vi "TestHarnessDPL-Saturday.vi"() -> ()   [LabVIEW 2024]
uses:
  <vilib>/Analysis/1siggen.llb/Ramp Pattern by Samples.vi
  <vilib>/measure/mamon.llb/Trigger Detection for 1 Channel.vi
  <vilib>/measure/mascope.llb/Transition Measurements 1 chan.vi
  <vilib>/Utility/file.llb/Write Delimited Spreadsheet (DBL).vi
  <vilib>/Analysis/1siggen.llb/Ramp Pattern by Delta.vi
  <vilib>/measure/mascope.llb/Amplitude and Levels 1 chan.vi
  <vilib>/Analysis/NI_AALBase.lvlib
  <userlib>/_OpenG.lib/time/time.llb/openg_time.lvlib
  <instrlib>/Detector SCPI/Detector SCPI.lvlib
  <instrlib>/Keithley 24XX/Keithley 24XX.lvlib
  <instrlib>/Keithley 648X Series/Keithley 648X Series.lvlib
  <vilib>/measure/NI_MAPro.lvlib
  <instrlib>/TTi TG5011a/TTi TG5011a.lvlib
panel:
  out "measurement info":T1 {"ref levels"."ref units" items=["absolute", "relative"]; "ref levels"."high ref level" format="%.2p"; "ref levels"."low ref level" format="%.2p"; "ref levels"."mid ref level" format="%.2p"; "end time" format="%.2p"; "start time" format="%.2p"}
  out "Searching":dbl[][](array[numeric])
  out "error out":errorcluster
  in  "Exit":bool
  in  "Measurement Mode":T2(tab)=enum."SweepCurrent (B2901)"
  in  "Heater":bool
  in  "DetectorData":T3(array[cluster])=[{"Name"="SWIR", "DAC Offset"=1870, "DAC StepsPerHGCount"=0.0}, {"Name"="MWIR", "DAC Offset"=688, "DAC StepsPerHGCount"=0.0}] {"DAC Offset" min=1 max=4095 step=1}
  in  "SPI Clock":i64=1000000
  in  "Oversample":i32=256 min=1 max=4096
  in  "Power":bool
  in  "Detector VISA":refnum<visa-resource-name>="Detector_EGSE"
  out "Detector Resource":refnum<visa-resource-name>="Detector_EGSE"
  out "Voltage (V)":dbl[](array[numeric])=[3.264, 0.0, 11.856, 11.996]
  out "Current (mA)":dbl[](array[numeric])=[0.0, 0.0, 12.8, -6.439]
  in  "ThrowAway":i32=100 min=1 max=10000
  out "Detector EGSE ID String":string="Aberystwyth University,Enfys Detector EGSE,#02.2,v0.5.0\r\n"
  in  "Current source":refnum<visa-resource-name>
  in  "Channel":i32 min=0 max=7
  in  "Collection":enum16{"Science", "Debug"}(ring)=enum."Debug"
  in  "Tolerance":dbl
  in  "Target Counts":i32 min=0 max=4095
  in  "Find Offset":bool
  out "Searching...":bool
  out "BoardTemperature":dbl=29.25
  in  "Tab Control":enum32{"Counts", "All Counts", "Temperature"}(tab)
  out "Counts":dbl(graph)=10.96875
  out "All Counts":T4(graph)={"subarray[0]"=1165.0625, "subarray[1]"=0.0, "subarray[2]"=4.4375, "subarray[3]"=4012.25, "subarray[4]"=2457.1875, "subarray[5]"=108.625, "subarray[6]"=1984.4375, "subarray[7]"=0.4375, "subarray[8]"=0.0}
  out "Temperature":dbl(graph)=29.25
  in  "ResetVDACstats":bool
  in  "Gain":u16(ring) items=["High", "Med", "Low"]
  in  "DAC Value":i32=688 min=0 max=4095 step=1
  in  "Detector":u16(ring)=1 items=["SWIR", "MWIR"]
  out "Peak-to-Peak (counts)":dbl=737.46875 format="%^.4g"
  out "rms (counts) 2":dbl=233.70780098659813 format="%^.4g"
  out "Mean Value (counts)":dbl=149.05195579441914
  out "Elapsed(uS)":i32=7203
  out "size":i32=439
  in  "Avg":i32=1 min=1 max=100
  in  "Pause":bool
  out "Waveform Graph":waveform(dbl)(graph)
  in  "Detector 3":u16(ring) items=["SWIR", "MWIR"]
  in  "Gain 3":u16(ring) items=["High", "Med", "Low"]
  in  "trigger slope":u16(ring)=1 items=["Falling Edge", "Rising Edge"]
  in  "level":dbl=2000.0 format="%#_13g"
  in  "hysteresis":dbl format="%.2p"
  out "Edge Time (ms)":dbl
  in  "SWIR/MWIR":bool=TRUE
  in  "SweepDataSelector":enum32{"Raw data", "SWIR"}(tab)
  in  "Export Button":bool
  out "Counts vs Channels":dbl[][](array[numeric])=[[1e-10, 128.75, 13.9375, 7.9375, 15.8125, 6.0, 7.25, 2030.9375, 4089.9375], [1.1220184543019634e-10, 129.9375, 14.0, 7.8125, 35.625, 6.0625, 7.1875, 2030.9375, 4089.9375], [1.2589254117941675e-10, 129.5, 13.9375, 8.0, 44.0625, 6.1875, 7.1875, 2030.9375, 4090.0], [1.4125375446227545e-10, 129.875, 14.0625, 7.9375, 17.3125, 6.125, 7.25, 2030.9375, 4089.875], [1.5848931924611137e-10, 129.9375, 14.0, 7.9375, 47.125, 6.125, 7.25, 2030.9375, 4089.9375], [1.778279410038923e-10, 130.125, 14.0625, 7.875, 32.875, 5.875, 7.1875, 2030.9375, 4090.0], [1.9952623149688797e-10, 129.5, 13.875, 7.875, 19.5, 5.8125, 7.3125, 2030.9375, 4089.9375], [2.23872113856834e-10, 130.0625, 13.9375, 7.9375, 12.625, 5.5625, 7.25, 2030.9375, 4090.0], [2.5118864315095804e-10, 130.8125, 14.0625, 7.9375, 20.3125, 6.0, 7.1875, 2030.9375, 4089.9375], [2.8183829312644536e-10, 129.75, 13.9375, 7.9375, 62.625, 6.25, 7.25, 2030.9375, 4089.9375], [3.1622776601683795e-10, 130.4375, 14.125, 7.9375, 53.75, 6.125, 7.25, 2030.9375, 4090.0], [3.5481338923357554e-10, 130.3125, 13.9375, 7.9375, 38.75, 5.9375, 7.1875, 2030.9375, 4089.875], [3.9810717055349735e-10, 129.8125, 14.0, 7.875, 45.75, 6.1875, 7.25, 2030.9375, 4090.0], [4.466835921509632e-10, 130.0, 14.0, 7.875, 76.4375, 6.4375, 7.25, 2030.9375, 4090.0], [5.011872336272724e-10, 130.625, 14.0625, 7.9375, 206.875, 9.25, 7.3125, 2030.9375, 4090.0], [5.623413251903491e-10, 130.3125, 13.9375, 7.875, 198.5, 8.9375, 7.25, 2030.9375, 4090.0], [6.309573444801933e-10, 130.0, 14.0625, 7.9375, 198.5625, 8.25, 7.25, 2030.9375, 4090.0], [7.07945784384138e-10, 130.5625, 14.125, 7.9375, 208.125, 8.4375, 7.3125, 2030.9375, 4089.875], [7.943282347242817e-10, 130.125, 13.9375, 7.875, 217.4375, 8.6875, 7.3125, 2030.9375, 4090.0], [8.912509381337457e-10, 130.0625, 13.9375, 7.9375, 206.875, 8.5625, 7.3125, 2030.9375, 4090.0], [1e-09, 129.9375, 13.9375, 7.875, 207.0, 8.4375, 7.375, 2030.9375, 4089.875], [1.1220184543019634e-09, 129.5, 13.9375, 7.875, 175.625, 8.125, 7.3125, 2030.9375, 4089.9375], [1.2589254117941673e-09, 130.75, 14.0, 7.875, 161.0, 7.9375, 7.3125, 2030.9375, 4090.0], [1.4125375446227544e-09, 130.0625, 14.0, 7.9375, 154.125, 7.75, 7.25, 2030.9375, 4089.9375], [1.5848931924611136e-09, 130.1875, 14.0, 7.875, 301.75, 10.5625, 7.375, 2030.9375, 4089.9375], [1.7782794100389228e-09, 130.875, 14.0625, 7.9375, 313.75, 10.8125, 7.4375, 2030.9375, 4089.875], [1.99526231496888e-09, 129.9375, 14.0, 7.8125, 299.75, 10.6875, 7.3125, 2030.9375, 4089.9375], [2.2387211385683402e-09, 129.875, 13.9375, 7.875, 298.1875, 10.375, 7.4375, 2030.9375, 4089.9375], [2.5118864315095803e-09, 130.75, 14.0, 7.9375, 441.125, 12.625, 7.375, 2030.875, 4090.0], [2.818382931264454e-09, 130.625, 14.0, 7.875, 490.4375, 13.375, 7.5, 2030.9375, 4089.9375], [3.1622776601683795e-09, 131.4375, 14.0625, 7.9375, 501.8125, 13.5625, 7.5, 2030.9375, 4090.0], [3.548133892335755e-09, 130.25, 14.0, 7.9375, 617.5, 15.3125, 7.625, 2030.9375, 4089.875], [3.981071705534974e-09, 129.6875, 13.9375, 7.875, 619.4375, 15.25, 7.5625, 2030.9375, 4090.0], [4.466835921509632e-09, 130.5, 14.0625, 7.875, 629.6875, 15.5, 7.5, 2030.9375, 4089.875], [5.011872336272724e-09, 130.875, 13.9375, 7.9375, 780.5625, 17.875, 7.5625, 2030.9375, 4090.0], [5.623413251903492e-09, 130.25, 14.125, 7.875, 917.1875, 20.125, 7.75, 2030.9375, 4090.0], [6.309573444801934e-09, 130.25, 14.0, 7.875, 931.5, 20.0625, 7.6875, 2030.9375, 4089.9375], [7.079457843841381e-09, 130.0, 14.0, 7.875, 1056.8125, 22.75, 7.8125, 2030.9375, 4090.0], [7.943282347242815e-09, 130.5625, 14.0625, 7.875, 1224.5, 24.8125, 7.8125, 2030.9375, 4090.0], [8.912509381337456e-09, 130.25, 14.0, 7.9375, 1380.75, 27.9375, 7.875, 2030.9375, 4089.9375], [1e-08, 130.125, 14.0, 7.9375, 1513.625, 29.9375, 8.0625, 2030.9375, 4089.875], [1.1220184543019634e-08, 130.625, 14.0, 7.9375, 1648.5, 34.5625, 8.125, 2030.9375, 4089.9375], [1.2589254117941673e-08, 131.0, 14.0625, 7.875, 1962.25, 41.625, 8.25, 2030.9375, 4090.0], [1.4125375446227542e-08, 130.875, 14.0625, 7.875, 2069.75, 44.625, 8.3125, 2030.9375, 4089.875], [1.5848931924611136e-08, 130.8125, 14.0625, 7.9375, 2404.875, 49.0, 8.4375, 2030.9375, 4089.9375], [1.7782794100389228e-08, 130.75, 14.125, 8.0, 2633.3125, 53.625, 8.6875, 2030.9375, 4090.125], [1.99526231496888e-08, 130.25, 14.0, 7.9375, 2979.375, 58.5, 8.8125, 2030.9375, 4090.0625], [2.2387211385683398e-08, 131.125, 14.0625, 7.9375, 3271.5, 64.5625, 8.9375, 2030.9375, 4089.9375], [2.51188643150958e-08, 131.4375, 14.125, 7.9375, 3737.375, 71.875, 9.25, 2030.9375, 4090.0], [2.8183829312644537e-08, 130.625, 14.0625, 7.875, 3908.375, 79.4375, 9.375, 2030.9375, 4089.9375], [3.16227766016838e-08, 130.875, 14.125, 7.8125, 3950.875, 88.5, 9.8125, 2030.9375, 4090.0625], [3.548133892335755e-08, 130.125, 14.0, 7.9375, 3963.5, 96.9375, 10.0, 2030.9375, 4090.0], [3.9810717055349736e-08, 130.375, 14.0, 7.875, 3980.25, 112.625, 10.25, 2030.9375, 4090.0625], [4.466835921509632e-08, 129.875, 14.0, 7.9375, 3991.125, 124.875, 10.6875, 2030.9375, 4090.0625], [5.0118723362727236e-08, 130.875, 14.0, 7.875, 3999.1875, 133.75, 11.1875, 2030.9375, 4090.0625], [5.623413251903492e-08, 130.25, 14.0, 8.0, 4007.9375, 147.125, 11.625, 2030.9375, 4090.0625], [6.309573444801934e-08, 130.75, 14.0625, 7.875, 4009.875, 168.1875, 12.1875, 2030.9375, 4090.0], [7.079457843841381e-08, 130.125, 13.9375, 7.875, 4010.0625, 187.6875, 12.875, 2030.9375, 4090.0], [7.943282347242817e-08, 130.1875, 14.0625, 7.9375, 4009.9375, 208.0625, 13.5625, 2030.9375, 4090.0], [8.912509381337456e-08, 130.75, 14.0625, 7.9375, 4010.0, 236.8125, 14.3125, 2030.9375, 4090.0], [1.0000000000000001e-07, 130.0, 14.0, 7.9375, 4010.0, 259.6875, 15.125, 2030.9375, 4089.9375], [1.1220184543019634e-07, 130.625, 14.125, 7.875, 4010.0, 288.4375, 16.125, 2030.9375, 4090.0625], [1.2589254117941672e-07, 130.6875, 14.0625, 8.0, 4009.9375, 326.375, 17.125, 2030.9375, 4090.0], [1.4125375446227544e-07, 130.5625, 14.0, 7.9375, 4010.0, 367.5625, 18.25, 2030.9375, 4090.0625], [1.5848931924611136e-07, 131.5, 14.0625, 7.875, 4010.0, 403.6875, 19.5, 2030.9375, 4090.0], [1.778279410038923e-07, 130.375, 14.0625, 7.9375, 4010.0, 457.875, 21.1875, 2030.9375, 4090.0], [1.9952623149688798e-07, 130.5625, 14.0, 8.0, 4010.0625, 512.6875, 22.875, 2030.9375, 4089.9375], [2.23872113856834e-07, 130.8125, 14.125, 7.9375, 4009.875, 571.875, 24.8125, 2030.9375, 4090.0], [2.51188643150958e-07, 130.125, 14.0, 7.9375, 4010.0625, 640.375, 26.9375, 2030.9375, 4090.125], [2.818382931264454e-07, 130.375, 14.0, 7.9375, 4010.0, 718.0625, 29.8125, 2030.9375, 4090.0], [3.1622776601683797e-07, 130.1875, 14.0625, 8.0, 4009.9375, 802.625, 34.125, 2030.9375, 4090.0625], [3.548133892335755e-07, 130.75, 14.0625, 7.9375, 4009.9375, 901.25, 39.375, 2030.9375, 4090.0625], [3.9810717055349735e-07, 130.4375, 14.0625, 7.9375, 4009.9375, 1014.0625, 43.8125, 2030.9375, 4089.9375], [4.4668359215096317e-07, 130.75, 14.125, 7.9375, 4009.8125, 1135.1875, 47.6875, 2030.9375, 4090.125], [5.011872336272724e-07, 130.5, 14.0625, 8.0, 4009.8125, 1270.3125, 52.0, 2030.9375, 4090.0625], [5.623413251903491e-07, 131.1875, 14.125, 7.9375, 4009.9375, 1418.75, 56.8125, 2030.9375, 4090.0], [6.309573444801933e-07, 130.625, 14.0, 7.9375, 4009.9375, 1591.875, 62.625, 2030.9375, 4090.0625], [7.07945784384138e-07, 130.25, 14.125, 7.9375, 4010.0, 1787.8125, 69.3125, 2031.0, 4090.0], [7.943282347242816e-07, 130.0625, 13.9375, 7.875, 4009.9375, 2000.625, 76.375, 2030.9375, 4090.0], [8.912509381337455e-07, 130.3125, 14.0625, 8.0625, 4009.8125, 2242.3125, 83.8125, 2030.9375, 4090.0625], [1e-06, 130.875, 14.0625, 7.9375, 4010.0, 2513.625, 92.6875, 2030.9375, 4090.0625], [1.1220184543019635e-06, 129.5625, 14.0, 8.0, 4009.8125, 2816.8125, 107.0, 2030.9375, 4090.0625], [1.2589254117941674e-06, 129.75, 14.0625, 7.9375, 4009.8125, 3157.6875, 118.25, 2030.9375, 4090.125], [1.4125375446227546e-06, 130.875, 14.0625, 7.875, 4009.9375, 3544.25, 128.75, 2030.9375, 4090.0625], [1.5848931924611137e-06, 130.125, 14.0625, 7.9375, 4009.9375, 3876.875, 140.5, 2030.9375, 4090.125], [1.7782794100389227e-06, 130.3125, 14.0625, 7.9375, 4009.75, 3932.25, 155.6875, 2030.9375, 4090.0], [1.9952623149688796e-06, 130.8125, 14.0625, 7.9375, 4009.75, 3955.5625, 177.8125, 2030.9375, 4090.1875], [2.23872113856834e-06, 129.9375, 14.0625, 8.0, 4009.875, 3970.6875, 198.0, 2030.9375, 4090.1875], [2.51188643150958e-06, 131.25, 14.1875, 8.0, 4009.875, 3982.125, 219.625, 2030.9375, 4090.125], [2.818382931264454e-06, 131.0, 14.125, 8.0, 4009.8125, 3992.0, 248.8125, 2030.9375, 4090.125], [3.1622776601683796e-06, 131.125, 14.0625, 8.0, 4009.9375, 4000.375, 272.8125, 2030.9375, 4090.0625], [3.548133892335755e-06, 131.3125, 14.125, 7.875, 4009.9375, 4006.3125, 308.25, 2030.9375, 4090.125], [3.981071705534973e-06, 130.875, 14.125, 7.9375, 4009.8125, 4006.3125, 343.3125, 2030.9375, 4090.1875], [4.466835921509632e-06, 130.5625, 14.125, 8.0, 4009.75, 4006.375, 385.0, 2030.9375, 4090.1875], [5.011872336272724e-06, 130.4375, 14.125, 8.0, 4009.875, 4006.3125, 431.1875, 2030.9375, 4090.1875], [5.623413251903491e-06, 130.25, 14.0625, 7.9375, 4010.0, 4006.3125, 481.875, 2030.9375, 4090.1875], [6.309573444801934e-06, 130.4375, 14.0625, 7.9375, 4009.9375, 4006.3125, 534.375, 2030.9375, 4090.125], [7.079457843841381e-06, 130.6875, 14.0625, 7.9375, 4009.875, 4006.3125, 601.1875, 2030.9375, 4090.125], [7.943282347242817e-06, 130.8125, 14.25, 8.0, 4009.875, 4006.3125, 671.5625, 2030.9375, 4090.1875], [8.912509381337456e-06, 130.6875, 14.0625, 8.0625, 4009.875, 4006.3125, 758.5, 2030.9375, 4090.125], [1e-05, 130.8125, 14.125, 8.0, 4009.75, 4006.3125, 847.125, 2030.9375, 4090.1875], [1.1220184543019633e-05, 131.25, 14.125, 8.0, 4009.8125, 4006.3125, 949.8125, 2030.9375, 4090.1875], [1.2589254117941673e-05, 130.625, 14.1875, 8.0, 4009.8125, 4006.3125, 1062.1875, 2030.9375, 4090.125], [1.4125375446227545e-05, 130.1875, 14.0625, 8.0, 4009.75, 4006.25, 1190.75, 2030.9375, 4090.1875], [1.5848931924611134e-05, 130.3125, 14.0625, 8.0, 4009.8125, 4006.3125, 1334.4375, 2030.9375, 4090.125], [1.778279410038923e-05, 130.625, 14.0625, 8.0, 4009.75, 4006.375, 1494.75, 2030.9375, 4090.1875], [1.99526231496888e-05, 130.75, 14.125, 8.0, 4009.8125, 4006.3125, 1672.4375, 2030.9375, 4090.25], [2.23872113856834e-05, 130.6875, 14.125, 8.0625, 4009.6875, 4006.375, 1877.3125, 2030.9375, 4090.25], [2.51188643150958e-05, 131.625, 14.1875, 8.0625, 4009.6875, 4006.3125, 2102.375, 2030.9375, 4090.1875], [2.818382931264454e-05, 129.875, 14.0625, 7.9375, 4009.75, 4006.25, 2358.0, 2030.9375, 4090.1875], [3.1622776601683795e-05, 130.1875, 14.125, 8.0, 4009.8125, 4006.3125, 2641.8125, 2030.9375, 4090.125], [3.5481338923357554e-05, 130.4375, 14.125, 8.0, 4009.75, 4006.375, 2960.6875, 2030.9375, 4090.1875], [3.9810717055349735e-05, 130.6875, 14.1875, 8.0, 4009.75, 4006.375, 3322.5, 2030.9375, 4090.125], [4.466835921509632e-05, 131.0, 14.125, 8.0, 4009.6875, 4006.375, 3719.875, 2031.0, 4090.1875], [5.011872336272724e-05, 130.75, 14.125, 8.0625, 4009.6875, 4006.375, 3911.125, 2030.9375, 4090.3125], [5.6234132519034914e-05, 130.875, 14.1875, 8.0625, 4009.625, 4006.375, 3946.3125, 2030.9375, 4090.25], [6.309573444801933e-05, 132.375, 14.1875, 8.0, 4009.625, 4006.3125, 3965.4375, 2031.0, 4090.3125], [7.079457843841381e-05, 131.1875, 14.25, 8.0, 4009.6875, 4006.375, 3979.0, 2030.9375, 4090.1875], [7.943282347242817e-05, 130.9375, 14.25, 8.0, 4009.625, 4006.375, 3990.25, 2031.0, 4090.1875], [8.912509381337456e-05, 130.9375, 14.25, 8.0625, 4009.5625, 4006.4375, 3999.8125, 2031.0, 4090.3125]]
  out "All Channel Data":cluster{dbl[], "output array":dbl[]}[](graph)=[{[1e-10, 1.1220184543019634e-10, 1.2589254117941675e-10, 1.4125375446227545e-10, 1.5848931924611137e-10, 1.778279410038923e-10, 1.9952623149688797e-10, 2.23872113856834e-10, 2.5118864315095804e-10, 2.8183829312644536e-10, 3.1622776601683795e-10, 3.5481338923357554e-10, 3.9810717055349735e-10, 4.466835921509632e-10, 5.011872336272724e-10, 5.623413251903491e-10, 6.309573444801933e-10, 7.07945784384138e-10, 7.943282347242817e-10, 8.912509381337457e-10, 1e-09, 1.1220184543019634e-09, 1.2589254117941673e-09, 1.4125375446227544e-09, 1.5848931924611136e-09, 1.7782794100389228e-09, 1.99526231496888e-09, 2.2387211385683402e-09, 2.5118864315095803e-09, 2.818382931264454e-09, 3.1622776601683795e-09, 3.548133892335755e-09, 3.981071705534974e-09, 4.466835921509632e-09, 5.011872336272724e-09, 5.623413251903492e-09, 6.309573444801934e-09, 7.079457843841381e-09, 7.943282347242815e-09, 8.912509381337456e-09, 1e-08, 1.1220184543019634e-08, 1.2589254117941673e-08, 1.4125375446227542e-08, 1.5848931924611136e-08, 1.7782794100389228e-08, 1.99526231496888e-08, 2.2387211385683398e-08, 2.51188643150958e-08, 2.8183829312644537e-08, 3.16227766016838e-08, 3.548133892335755e-08, 3.9810717055349736e-08, 4.466835921509632e-08, 5.0118723362727236e-08, 5.623413251903492e-08, 6.309573444801934e-08, 7.079457843841381e-08, 7.943282347242817e-08, 8.912509381337456e-08, 1.0000000000000001e-07, 1.1220184543019634e-07, 1.2589254117941672e-07, 1.4125375446227544e-07, 1.5848931924611136e-07, 1.778279410038923e-07, 1.9952623149688798e-07, 2.23872113856834e-07, 2.51188643150958e-07, 2.818382931264454e-07, 3.1622776601683797e-07, 3.548133892335755e-07, 3.9810717055349735e-07, 4.4668359215096317e-07, 5.011872336272724e-07, 5.623413251903491e-07, 6.309573444801933e-07, 7.07945784384138e-07, 7.943282347242816e-07, 8.912509381337455e-07, 1e-06, 1.1220184543019635e-06, 1.2589254117941674e-06, 1.4125375446227546e-06, 1.5848931924611137e-06, 1.7782794100389227e-06, 1.9952623149688796e-06, 2.23872113856834e-06, 2.51188643150958e-06, 2.818382931264454e-06, 3.1622776601683796e-06, 3.548133892335755e-06, 3.981071705534973e-06, 4.466835921509632e-06, 5.011872336272724e-06, 5.623413251903491e-06, 6.309573444801934e-06, 7.079457843841381e-06, 7.943282347242817e-06, 8.912509381337456e-06, 1e-05, 1.1220184543019633e-05, 1.2589254117941673e-05, 1.4125375446227545e-05, 1.5848931924611134e-05, 1.778279410038923e-05, 1.99526231496888e-05, 2.23872113856834e-05, 2.51188643150958e-05, 2.818382931264454e-05, 3.1622776601683795e-05, 3.5481338923357554e-05, 3.9810717055349735e-05, 4.466835921509632e-05, 5.011872336272724e-05, 5.6234132519034914e-05, 6.309573444801933e-05, 7.079457843841381e-05, 7.943282347242817e-05, 8.912509381337456e-05], "output array"=[15.8125, 35.625, 44.0625, 17.3125, 47.125, 32.875, 19.5, 12.625, 20.3125, 62.625, 53.75, 38.75, 45.75, 76.4375, 206.875, 198.5, 198.5625, 208.125, 217.4375, 206.875, 207.0, 175.625, 161.0, 154.125, 301.75, 313.75, 299.75, 298.1875, 441.125, 490.4375, 501.8125, 617.5, 619.4375, 629.6875, 780.5625, 917.1875, 931.5, 1056.8125, 1224.5, 1380.75, 1513.625, 1648.5, 1962.25, 2069.75, 2404.875, 2633.3125, 2979.375, 3271.5, 3737.375, 3908.375, 3950.875, 3963.5, 3980.25, 3991.125, 3999.1875, 4007.9375, 4009.875, 4010.0625, 4009.9375, 4010.0, 4010.0, 4010.0, 4009.9375, 4010.0, 4010.0, 4010.0, 4010.0625, 4009.875, 4010.0625, 4010.0, 4009.9375, 4009.9375, 4009.9375, 4009.8125, 4009.8125, 4009.9375, 4009.9375, 4010.0, 4009.9375, 4009.8125, 4010.0, 4009.8125, 4009.8125, 4009.9375, 4009.9375, 4009.75, 4009.75, 4009.875, 4009.875, 4009.8125, 4009.9375, 4009.9375, 4009.8125, 4009.75, 4009.875, 4010.0, 4009.9375, 4009.875, 4009.875, 4009.875, 4009.75, 4009.8125, 4009.8125, 4009.75, 4009.8125, 4009.75, 4009.8125, 4009.6875, 4009.6875, 4009.75, 4009.8125, 4009.75, 4009.75, 4009.6875, 4009.6875, 4009.625, 4009.625, 4009.6875, 4009.625, 4009.5625]}, {[1e-10, 1.1220184543019634e-10, 1.2589254117941675e-10, 1.4125375446227545e-10, 1.5848931924611137e-10, 1.778279410038923e-10, 1.9952623149688797e-10, 2.23872113856834e-10, 2.5118864315095804e-10, 2.8183829312644536e-10, 3.1622776601683795e-10, 3.5481338923357554e-10, 3.9810717055349735e-10, 4.466835921509632e-10, 5.011872336272724e-10, 5.623413251903491e-10, 6.309573444801933e-10, 7.07945784384138e-10, 7.943282347242817e-10, 8.912509381337457e-10, 1e-09, 1.1220184543019634e-09, 1.2589254117941673e-09, 1.4125375446227544e-09, 1.5848931924611136e-09, 1.7782794100389228e-09, 1.99526231496888e-09, 2.2387211385683402e-09, 2.5118864315095803e-09, 2.818382931264454e-09, 3.1622776601683795e-09, 3.548133892335755e-09, 3.981071705534974e-09, 4.466835921509632e-09, 5.011872336272724e-09, 5.623413251903492e-09, 6.309573444801934e-09, 7.079457843841381e-09, 7.943282347242815e-09, 8.912509381337456e-09, 1e-08, 1.1220184543019634e-08, 1.2589254117941673e-08, 1.4125375446227542e-08, 1.5848931924611136e-08, 1.7782794100389228e-08, 1.99526231496888e-08, 2.2387211385683398e-08, 2.51188643150958e-08, 2.8183829312644537e-08, 3.16227766016838e-08, 3.548133892335755e-08, 3.9810717055349736e-08, 4.466835921509632e-08, 5.0118723362727236e-08, 5.623413251903492e-08, 6.309573444801934e-08, 7.079457843841381e-08, 7.943282347242817e-08, 8.912509381337456e-08, 1.0000000000000001e-07, 1.1220184543019634e-07, 1.2589254117941672e-07, 1.4125375446227544e-07, 1.5848931924611136e-07, 1.778279410038923e-07, 1.9952623149688798e-07, 2.23872113856834e-07, 2.51188643150958e-07, 2.818382931264454e-07, 3.1622776601683797e-07, 3.548133892335755e-07, 3.9810717055349735e-07, 4.4668359215096317e-07, 5.011872336272724e-07, 5.623413251903491e-07, 6.309573444801933e-07, 7.07945784384138e-07, 7.943282347242816e-07, 8.912509381337455e-07, 1e-06, 1.1220184543019635e-06, 1.2589254117941674e-06, 1.4125375446227546e-06, 1.5848931924611137e-06, 1.7782794100389227e-06, 1.9952623149688796e-06, 2.23872113856834e-06, 2.51188643150958e-06, 2.818382931264454e-06, 3.1622776601683796e-06, 3.548133892335755e-06, 3.981071705534973e-06, 4.466835921509632e-06, 5.011872336272724e-06, 5.623413251903491e-06, 6.309573444801934e-06, 7.079457843841381e-06, 7.943282347242817e-06, 8.912509381337456e-06, 1e-05, 1.1220184543019633e-05, 1.2589254117941673e-05, 1.4125375446227545e-05, 1.5848931924611134e-05, 1.778279410038923e-05, 1.99526231496888e-05, 2.23872113856834e-05, 2.51188643150958e-05, 2.818382931264454e-05, 3.1622776601683795e-05, 3.5481338923357554e-05, 3.9810717055349735e-05, 4.466835921509632e-05, 5.011872336272724e-05, 5.6234132519034914e-05, 6.309573444801933e-05, 7.079457843841381e-05, 7.943282347242817e-05, 8.912509381337456e-05], "output array"=[6.0, 6.0625, 6.1875, 6.125, 6.125, 5.875, 5.8125, 5.5625, 6.0, 6.25, 6.125, 5.9375, 6.1875, 6.4375, 9.25, 8.9375, 8.25, 8.4375, 8.6875, 8.5625, 8.4375, 8.125, 7.9375, 7.75, 10.5625, 10.8125, 10.6875, 10.375, 12.625, 13.375, 13.5625, 15.3125, 15.25, 15.5, 17.875, 20.125, 20.0625, 22.75, 24.8125, 27.9375, 29.9375, 34.5625, 41.625, 44.625, 49.0, 53.625, 58.5, 64.5625, 71.875, 79.4375, 88.5, 96.9375, 112.625, 124.875, 133.75, 147.125, 168.1875, 187.6875, 208.0625, 236.8125, 259.6875, 288.4375, 326.375, 367.5625, 403.6875, 457.875, 512.6875, 571.875, 640.375, 718.0625, 802.625, 901.25, 1014.0625, 1135.1875, 1270.3125, 1418.75, 1591.875, 1787.8125, 2000.625, 2242.3125, 2513.625, 2816.8125, 3157.6875, 3544.25, 3876.875, 3932.25, 3955.5625, 3970.6875, 3982.125, 3992.0, 4000.375, 4006.3125, 4006.3125, 4006.375, 4006.3125, 4006.3125, 4006.3125, 4006.3125, 4006.3125, 4006.3125, 4006.3125, 4006.3125, 4006.3125, 4006.25, 4006.3125, 4006.375, 4006.3125, 4006.375, 4006.3125, 4006.25, 4006.3125, 4006.375, 4006.375, 4006.375, 4006.375, 4006.375, 4006.3125, 4006.375, 4006.375, 4006.4375]}, {[1e-10, 1.1220184543019634e-10, 1.2589254117941675e-10, 1.4125375446227545e-10, 1.5848931924611137e-10, 1.778279410038923e-10, 1.9952623149688797e-10, 2.23872113856834e-10, 2.5118864315095804e-10, 2.8183829312644536e-10, 3.1622776601683795e-10, 3.5481338923357554e-10, 3.9810717055349735e-10, 4.466835921509632e-10, 5.011872336272724e-10, 5.623413251903491e-10, 6.309573444801933e-10, 7.07945784384138e-10, 7.943282347242817e-10, 8.912509381337457e-10, 1e-09, 1.1220184543019634e-09, 1.2589254117941673e-09, 1.4125375446227544e-09, 1.5848931924611136e-09, 1.7782794100389228e-09, 1.99526231496888e-09, 2.2387211385683402e-09, 2.5118864315095803e-09, 2.818382931264454e-09, 3.1622776601683795e-09, 3.548133892335755e-09, 3.981071705534974e-09, 4.466835921509632e-09, 5.011872336272724e-09, 5.623413251903492e-09, 6.309573444801934e-09, 7.079457843841381e-09, 7.943282347242815e-09, 8.912509381337456e-09, 1e-08, 1.1220184543019634e-08, 1.2589254117941673e-08, 1.4125375446227542e-08, 1.5848931924611136e-08, 1.7782794100389228e-08, 1.99526231496888e-08, 2.2387211385683398e-08, 2.51188643150958e-08, 2.8183829312644537e-08, 3.16227766016838e-08, 3.548133892335755e-08, 3.9810717055349736e-08, 4.466835921509632e-08, 5.0118723362727236e-08, 5.623413251903492e-08, 6.309573444801934e-08, 7.079457843841381e-08, 7.943282347242817e-08, 8.912509381337456e-08, 1.0000000000000001e-07, 1.1220184543019634e-07, 1.2589254117941672e-07, 1.4125375446227544e-07, 1.5848931924611136e-07, 1.778279410038923e-07, 1.9952623149688798e-07, 2.23872113856834e-07, 2.51188643150958e-07, 2.818382931264454e-07, 3.1622776601683797e-07, 3.548133892335755e-07, 3.9810717055349735e-07, 4.4668359215096317e-07, 5.011872336272724e-07, 5.623413251903491e-07, 6.309573444801933e-07, 7.07945784384138e-07, 7.943282347242816e-07, 8.912509381337455e-07, 1e-06, 1.1220184543019635e-06, 1.2589254117941674e-06, 1.4125375446227546e-06, 1.5848931924611137e-06, 1.7782794100389227e-06, 1.9952623149688796e-06, 2.23872113856834e-06, 2.51188643150958e-06, 2.818382931264454e-06, 3.1622776601683796e-06, 3.548133892335755e-06, 3.981071705534973e-06, 4.466835921509632e-06, 5.011872336272724e-06, 5.623413251903491e-06, 6.309573444801934e-06, 7.079457843841381e-06, 7.943282347242817e-06, 8.912509381337456e-06, 1e-05, 1.1220184543019633e-05, 1.2589254117941673e-05, 1.4125375446227545e-05, 1.5848931924611134e-05, 1.778279410038923e-05, 1.99526231496888e-05, 2.23872113856834e-05, 2.51188643150958e-05, 2.818382931264454e-05, 3.1622776601683795e-05, 3.5481338923357554e-05, 3.9810717055349735e-05, 4.466835921509632e-05, 5.011872336272724e-05, 5.6234132519034914e-05, 6.309573444801933e-05, 7.079457843841381e-05, 7.943282347242817e-05, 8.912509381337456e-05], "output array"=[7.25, 7.1875, 7.1875, 7.25, 7.25, 7.1875, 7.3125, 7.25, 7.1875, 7.25, 7.25, 7.1875, 7.25, 7.25, 7.3125, 7.25, 7.25, 7.3125, 7.3125, 7.3125, 7.375, 7.3125, 7.3125, 7.25, 7.375, 7.4375, 7.3125, 7.4375, 7.375, 7.5, 7.5, 7.625, 7.5625, 7.5, 7.5625, 7.75, 7.6875, 7.8125, 7.8125, 7.875, 8.0625, 8.125, 8.25, 8.3125, 8.4375, 8.6875, 8.8125, 8.9375, 9.25, 9.375, 9.8125, 10.0, 10.25, 10.6875, 11.1875, 11.625, 12.1875, 12.875, 13.5625, 14.3125, 15.125, 16.125, 17.125, 18.25, 19.5, 21.1875, 22.875, 24.8125, 26.9375, 29.8125, 34.125, 39.375, 43.8125, 47.6875, 52.0, 56.8125, 62.625, 69.3125, 76.375, 83.8125, 92.6875, 107.0, 118.25, 128.75, 140.5, 155.6875, 177.8125, 198.0, 219.625, 248.8125, 272.8125, 308.25, 343.3125, 385.0, 431.1875, 481.875, 534.375, 601.1875, 671.5625, 758.5, 847.125, 949.8125, 1062.1875, 1190.75, 1334.4375, 1494.75, 1672.4375, 1877.3125, 2102.375, 2358.0, 2641.8125, 2960.6875, 3322.5, 3719.875, 3911.125, 3946.3125, 3965.4375, 3979.0, 3990.25, 3999.8125]}]
  in  "ISweep":bool
  in  "NPoints":i32=10 min=10 max=10000 step=1
  in  "MaxCurrent":dbl=1e-11 min=1e-11 max=1e-06
  in  "MinCurrent":dbl=1e-10 min=-10.0 max=10.0
  in  "DecadeSweep":bool=TRUE
  in  "milliseconds stabilisation":u32=10
  in  "SuperAverage":i32=1 min=1 max=100
  in  "NPointsPerDecade":u16(ring)=3 items=["1", "3", "9", "20"]
  in  "Tab Control 2":enum32{"Raw Data", "Plot"}(tab)
  in  "ExportData":bool
  out "Counts vs Channels 2":dbl[][](array[numeric])=[[1e-10, 128.75, 13.9375, 7.9375, 15.8125, 6.0, 7.25, 2030.9375, 4089.9375], [1.1220184543019634e-10, 129.9375, 14.0, 7.8125, 35.625, 6.0625, 7.1875, 2030.9375, 4089.9375], [1.2589254117941675e-10, 129.5, 13.9375, 8.0, 44.0625, 6.1875, 7.1875, 2030.9375, 4090.0], [1.4125375446227545e-10, 129.875, 14.0625, 7.9375, 17.3125, 6.125, 7.25, 2030.9375, 4089.875], [1.5848931924611137e-10, 129.9375, 14.0, 7.9375, 47.125, 6.125, 7.25, 2030.9375, 4089.9375], [1.778279410038923e-10, 130.125, 14.0625, 7.875, 32.875, 5.875, 7.1875, 2030.9375, 4090.0], [1.9952623149688797e-10, 129.5, 13.875, 7.875, 19.5, 5.8125, 7.3125, 2030.9375, 4089.9375], [2.23872113856834e-10, 130.0625, 13.9375, 7.9375, 12.625, 5.5625, 7.25, 2030.9375, 4090.0], [2.5118864315095804e-10, 130.8125, 14.0625, 7.9375, 20.3125, 6.0, 7.1875, 2030.9375, 4089.9375], [2.8183829312644536e-10, 129.75, 13.9375, 7.9375, 62.625, 6.25, 7.25, 2030.9375, 4089.9375], [3.1622776601683795e-10, 130.4375, 14.125, 7.9375, 53.75, 6.125, 7.25, 2030.9375, 4090.0], [3.5481338923357554e-10, 130.3125, 13.9375, 7.9375, 38.75, 5.9375, 7.1875, 2030.9375, 4089.875], [3.9810717055349735e-10, 129.8125, 14.0, 7.875, 45.75, 6.1875, 7.25, 2030.9375, 4090.0], [4.466835921509632e-10, 130.0, 14.0, 7.875, 76.4375, 6.4375, 7.25, 2030.9375, 4090.0], [5.011872336272724e-10, 130.625, 14.0625, 7.9375, 206.875, 9.25, 7.3125, 2030.9375, 4090.0], [5.623413251903491e-10, 130.3125, 13.9375, 7.875, 198.5, 8.9375, 7.25, 2030.9375, 4090.0], [6.309573444801933e-10, 130.0, 14.0625, 7.9375, 198.5625, 8.25, 7.25, 2030.9375, 4090.0], [7.07945784384138e-10, 130.5625, 14.125, 7.9375, 208.125, 8.4375, 7.3125, 2030.9375, 4089.875], [7.943282347242817e-10, 130.125, 13.9375, 7.875, 217.4375, 8.6875, 7.3125, 2030.9375, 4090.0], [8.912509381337457e-10, 130.0625, 13.9375, 7.9375, 206.875, 8.5625, 7.3125, 2030.9375, 4090.0], [1e-09, 129.9375, 13.9375, 7.875, 207.0, 8.4375, 7.375, 2030.9375, 4089.875], [1.1220184543019634e-09, 129.5, 13.9375, 7.875, 175.625, 8.125, 7.3125, 2030.9375, 4089.9375], [1.2589254117941673e-09, 130.75, 14.0, 7.875, 161.0, 7.9375, 7.3125, 2030.9375, 4090.0], [1.4125375446227544e-09, 130.0625, 14.0, 7.9375, 154.125, 7.75, 7.25, 2030.9375, 4089.9375], [1.5848931924611136e-09, 130.1875, 14.0, 7.875, 301.75, 10.5625, 7.375, 2030.9375, 4089.9375], [1.7782794100389228e-09, 130.875, 14.0625, 7.9375, 313.75, 10.8125, 7.4375, 2030.9375, 4089.875], [1.99526231496888e-09, 129.9375, 14.0, 7.8125, 299.75, 10.6875, 7.3125, 2030.9375, 4089.9375], [2.2387211385683402e-09, 129.875, 13.9375, 7.875, 298.1875, 10.375, 7.4375, 2030.9375, 4089.9375], [2.5118864315095803e-09, 130.75, 14.0, 7.9375, 441.125, 12.625, 7.375, 2030.875, 4090.0], [2.818382931264454e-09, 130.625, 14.0, 7.875, 490.4375, 13.375, 7.5, 2030.9375, 4089.9375], [3.1622776601683795e-09, 131.4375, 14.0625, 7.9375, 501.8125, 13.5625, 7.5, 2030.9375, 4090.0], [3.548133892335755e-09, 130.25, 14.0, 7.9375, 617.5, 15.3125, 7.625, 2030.9375, 4089.875], [3.981071705534974e-09, 129.6875, 13.9375, 7.875, 619.4375, 15.25, 7.5625, 2030.9375, 4090.0], [4.466835921509632e-09, 130.5, 14.0625, 7.875, 629.6875, 15.5, 7.5, 2030.9375, 4089.875], [5.011872336272724e-09, 130.875, 13.9375, 7.9375, 780.5625, 17.875, 7.5625, 2030.9375, 4090.0], [5.623413251903492e-09, 130.25, 14.125, 7.875, 917.1875, 20.125, 7.75, 2030.9375, 4090.0], [6.309573444801934e-09, 130.25, 14.0, 7.875, 931.5, 20.0625, 7.6875, 2030.9375, 4089.9375], [7.079457843841381e-09, 130.0, 14.0, 7.875, 1056.8125, 22.75, 7.8125, 2030.9375, 4090.0], [7.943282347242815e-09, 130.5625, 14.0625, 7.875, 1224.5, 24.8125, 7.8125, 2030.9375, 4090.0], [8.912509381337456e-09, 130.25, 14.0, 7.9375, 1380.75, 27.9375, 7.875, 2030.9375, 4089.9375], [1e-08, 130.125, 14.0, 7.9375, 1513.625, 29.9375, 8.0625, 2030.9375, 4089.875], [1.1220184543019634e-08, 130.625, 14.0, 7.9375, 1648.5, 34.5625, 8.125, 2030.9375, 4089.9375], [1.2589254117941673e-08, 131.0, 14.0625, 7.875, 1962.25, 41.625, 8.25, 2030.9375, 4090.0], [1.4125375446227542e-08, 130.875, 14.0625, 7.875, 2069.75, 44.625, 8.3125, 2030.9375, 4089.875], [1.5848931924611136e-08, 130.8125, 14.0625, 7.9375, 2404.875, 49.0, 8.4375, 2030.9375, 4089.9375], [1.7782794100389228e-08, 130.75, 14.125, 8.0, 2633.3125, 53.625, 8.6875, 2030.9375, 4090.125], [1.99526231496888e-08, 130.25, 14.0, 7.9375, 2979.375, 58.5, 8.8125, 2030.9375, 4090.0625], [2.2387211385683398e-08, 131.125, 14.0625, 7.9375, 3271.5, 64.5625, 8.9375, 2030.9375, 4089.9375], [2.51188643150958e-08, 131.4375, 14.125, 7.9375, 3737.375, 71.875, 9.25, 2030.9375, 4090.0], [2.8183829312644537e-08, 130.625, 14.0625, 7.875, 3908.375, 79.4375, 9.375, 2030.9375, 4089.9375], [3.16227766016838e-08, 130.875, 14.125, 7.8125, 3950.875, 88.5, 9.8125, 2030.9375, 4090.0625], [3.548133892335755e-08, 130.125, 14.0, 7.9375, 3963.5, 96.9375, 10.0, 2030.9375, 4090.0], [3.9810717055349736e-08, 130.375, 14.0, 7.875, 3980.25, 112.625, 10.25, 2030.9375, 4090.0625], [4.466835921509632e-08, 129.875, 14.0, 7.9375, 3991.125, 124.875, 10.6875, 2030.9375, 4090.0625], [5.0118723362727236e-08, 130.875, 14.0, 7.875, 3999.1875, 133.75, 11.1875, 2030.9375, 4090.0625], [5.623413251903492e-08, 130.25, 14.0, 8.0, 4007.9375, 147.125, 11.625, 2030.9375, 4090.0625], [6.309573444801934e-08, 130.75, 14.0625, 7.875, 4009.875, 168.1875, 12.1875, 2030.9375, 4090.0], [7.079457843841381e-08, 130.125, 13.9375, 7.875, 4010.0625, 187.6875, 12.875, 2030.9375, 4090.0], [7.943282347242817e-08, 130.1875, 14.0625, 7.9375, 4009.9375, 208.0625, 13.5625, 2030.9375, 4090.0], [8.912509381337456e-08, 130.75, 14.0625, 7.9375, 4010.0, 236.8125, 14.3125, 2030.9375, 4090.0], [1.0000000000000001e-07, 130.0, 14.0, 7.9375, 4010.0, 259.6875, 15.125, 2030.9375, 4089.9375], [1.1220184543019634e-07, 130.625, 14.125, 7.875, 4010.0, 288.4375, 16.125, 2030.9375, 4090.0625], [1.2589254117941672e-07, 130.6875, 14.0625, 8.0, 4009.9375, 326.375, 17.125, 2030.9375, 4090.0], [1.4125375446227544e-07, 130.5625, 14.0, 7.9375, 4010.0, 367.5625, 18.25, 2030.9375, 4090.0625], [1.5848931924611136e-07, 131.5, 14.0625, 7.875, 4010.0, 403.6875, 19.5, 2030.9375, 4090.0], [1.778279410038923e-07, 130.375, 14.0625, 7.9375, 4010.0, 457.875, 21.1875, 2030.9375, 4090.0], [1.9952623149688798e-07, 130.5625, 14.0, 8.0, 4010.0625, 512.6875, 22.875, 2030.9375, 4089.9375], [2.23872113856834e-07, 130.8125, 14.125, 7.9375, 4009.875, 571.875, 24.8125, 2030.9375, 4090.0], [2.51188643150958e-07, 130.125, 14.0, 7.9375, 4010.0625, 640.375, 26.9375, 2030.9375, 4090.125], [2.818382931264454e-07, 130.375, 14.0, 7.9375, 4010.0, 718.0625, 29.8125, 2030.9375, 4090.0], [3.1622776601683797e-07, 130.1875, 14.0625, 8.0, 4009.9375, 802.625, 34.125, 2030.9375, 4090.0625], [3.548133892335755e-07, 130.75, 14.0625, 7.9375, 4009.9375, 901.25, 39.375, 2030.9375, 4090.0625], [3.9810717055349735e-07, 130.4375, 14.0625, 7.9375, 4009.9375, 1014.0625, 43.8125, 2030.9375, 4089.9375], [4.4668359215096317e-07, 130.75, 14.125, 7.9375, 4009.8125, 1135.1875, 47.6875, 2030.9375, 4090.125], [5.011872336272724e-07, 130.5, 14.0625, 8.0, 4009.8125, 1270.3125, 52.0, 2030.9375, 4090.0625], [5.623413251903491e-07, 131.1875, 14.125, 7.9375, 4009.9375, 1418.75, 56.8125, 2030.9375, 4090.0], [6.309573444801933e-07, 130.625, 14.0, 7.9375, 4009.9375, 1591.875, 62.625, 2030.9375, 4090.0625], [7.07945784384138e-07, 130.25, 14.125, 7.9375, 4010.0, 1787.8125, 69.3125, 2031.0, 4090.0], [7.943282347242816e-07, 130.0625, 13.9375, 7.875, 4009.9375, 2000.625, 76.375, 2030.9375, 4090.0], [8.912509381337455e-07, 130.3125, 14.0625, 8.0625, 4009.8125, 2242.3125, 83.8125, 2030.9375, 4090.0625], [1e-06, 130.875, 14.0625, 7.9375, 4010.0, 2513.625, 92.6875, 2030.9375, 4090.0625], [1.1220184543019635e-06, 129.5625, 14.0, 8.0, 4009.8125, 2816.8125, 107.0, 2030.9375, 4090.0625], [1.2589254117941674e-06, 129.75, 14.0625, 7.9375, 4009.8125, 3157.6875, 118.25, 2030.9375, 4090.125], [1.4125375446227546e-06, 130.875, 14.0625, 7.875, 4009.9375, 3544.25, 128.75, 2030.9375, 4090.0625], [1.5848931924611137e-06, 130.125, 14.0625, 7.9375, 4009.9375, 3876.875, 140.5, 2030.9375, 4090.125], [1.7782794100389227e-06, 130.3125, 14.0625, 7.9375, 4009.75, 3932.25, 155.6875, 2030.9375, 4090.0], [1.9952623149688796e-06, 130.8125, 14.0625, 7.9375, 4009.75, 3955.5625, 177.8125, 2030.9375, 4090.1875], [2.23872113856834e-06, 129.9375, 14.0625, 8.0, 4009.875, 3970.6875, 198.0, 2030.9375, 4090.1875], [2.51188643150958e-06, 131.25, 14.1875, 8.0, 4009.875, 3982.125, 219.625, 2030.9375, 4090.125], [2.818382931264454e-06, 131.0, 14.125, 8.0, 4009.8125, 3992.0, 248.8125, 2030.9375, 4090.125], [3.1622776601683796e-06, 131.125, 14.0625, 8.0, 4009.9375, 4000.375, 272.8125, 2030.9375, 4090.0625], [3.548133892335755e-06, 131.3125, 14.125, 7.875, 4009.9375, 4006.3125, 308.25, 2030.9375, 4090.125], [3.981071705534973e-06, 130.875, 14.125, 7.9375, 4009.8125, 4006.3125, 343.3125, 2030.9375, 4090.1875], [4.466835921509632e-06, 130.5625, 14.125, 8.0, 4009.75, 4006.375, 385.0, 2030.9375, 4090.1875], [5.011872336272724e-06, 130.4375, 14.125, 8.0, 4009.875, 4006.3125, 431.1875, 2030.9375, 4090.1875], [5.623413251903491e-06, 130.25, 14.0625, 7.9375, 4010.0, 4006.3125, 481.875, 2030.9375, 4090.1875], [6.309573444801934e-06, 130.4375, 14.0625, 7.9375, 4009.9375, 4006.3125, 534.375, 2030.9375, 4090.125], [7.079457843841381e-06, 130.6875, 14.0625, 7.9375, 4009.875, 4006.3125, 601.1875, 2030.9375, 4090.125], [7.943282347242817e-06, 130.8125, 14.25, 8.0, 4009.875, 4006.3125, 671.5625, 2030.9375, 4090.1875], [8.912509381337456e-06, 130.6875, 14.0625, 8.0625, 4009.875, 4006.3125, 758.5, 2030.9375, 4090.125], [1e-05, 130.8125, 14.125, 8.0, 4009.75, 4006.3125, 847.125, 2030.9375, 4090.1875], [1.1220184543019633e-05, 131.25, 14.125, 8.0, 4009.8125, 4006.3125, 949.8125, 2030.9375, 4090.1875], [1.2589254117941673e-05, 130.625, 14.1875, 8.0, 4009.8125, 4006.3125, 1062.1875, 2030.9375, 4090.125], [1.4125375446227545e-05, 130.1875, 14.0625, 8.0, 4009.75, 4006.25, 1190.75, 2030.9375, 4090.1875], [1.5848931924611134e-05, 130.3125, 14.0625, 8.0, 4009.8125, 4006.3125, 1334.4375, 2030.9375, 4090.125], [1.778279410038923e-05, 130.625, 14.0625, 8.0, 4009.75, 4006.375, 1494.75, 2030.9375, 4090.1875], [1.99526231496888e-05, 130.75, 14.125, 8.0, 4009.8125, 4006.3125, 1672.4375, 2030.9375, 4090.25], [2.23872113856834e-05, 130.6875, 14.125, 8.0625, 4009.6875, 4006.375, 1877.3125, 2030.9375, 4090.25], [2.51188643150958e-05, 131.625, 14.1875, 8.0625, 4009.6875, 4006.3125, 2102.375, 2030.9375, 4090.1875], [2.818382931264454e-05, 129.875, 14.0625, 7.9375, 4009.75, 4006.25, 2358.0, 2030.9375, 4090.1875], [3.1622776601683795e-05, 130.1875, 14.125, 8.0, 4009.8125, 4006.3125, 2641.8125, 2030.9375, 4090.125], [3.5481338923357554e-05, 130.4375, 14.125, 8.0, 4009.75, 4006.375, 2960.6875, 2030.9375, 4090.1875], [3.9810717055349735e-05, 130.6875, 14.1875, 8.0, 4009.75, 4006.375, 3322.5, 2030.9375, 4090.125], [4.466835921509632e-05, 131.0, 14.125, 8.0, 4009.6875, 4006.375, 3719.875, 2031.0, 4090.1875], [5.011872336272724e-05, 130.75, 14.125, 8.0625, 4009.6875, 4006.375, 3911.125, 2030.9375, 4090.3125], [5.6234132519034914e-05, 130.875, 14.1875, 8.0625, 4009.625, 4006.375, 3946.3125, 2030.9375, 4090.25], [6.309573444801933e-05, 132.375, 14.1875, 8.0, 4009.625, 4006.3125, 3965.4375, 2031.0, 4090.3125], [7.079457843841381e-05, 131.1875, 14.25, 8.0, 4009.6875, 4006.375, 3979.0, 2030.9375, 4090.1875], [7.943282347242817e-05, 130.9375, 14.25, 8.0, 4009.625, 4006.375, 3990.25, 2031.0, 4090.1875], [8.912509381337456e-05, 130.9375, 14.25, 8.0625, 4009.5625, 4006.4375, 3999.8125, 2031.0, 4090.3125]]
  out "All Channel Data 2":cluster{dbl[], "output array":dbl[]}[](graph)=[{[1e-10, 1.1220184543019634e-10, 1.2589254117941675e-10, 1.4125375446227545e-10, 1.5848931924611137e-10, 1.778279410038923e-10, 1.9952623149688797e-10, 2.23872113856834e-10, 2.5118864315095804e-10, 2.8183829312644536e-10, 3.1622776601683795e-10, 3.5481338923357554e-10, 3.9810717055349735e-10, 4.466835921509632e-10, 5.011872336272724e-10, 5.623413251903491e-10, 6.309573444801933e-10, 7.07945784384138e-10, 7.943282347242817e-10, 8.912509381337457e-10, 1e-09, 1.1220184543019634e-09, 1.2589254117941673e-09, 1.4125375446227544e-09, 1.5848931924611136e-09, 1.7782794100389228e-09, 1.99526231496888e-09, 2.2387211385683402e-09, 2.5118864315095803e-09, 2.818382931264454e-09, 3.1622776601683795e-09, 3.548133892335755e-09, 3.981071705534974e-09, 4.466835921509632e-09, 5.011872336272724e-09, 5.623413251903492e-09, 6.309573444801934e-09, 7.079457843841381e-09, 7.943282347242815e-09, 8.912509381337456e-09, 1e-08, 1.1220184543019634e-08, 1.2589254117941673e-08, 1.4125375446227542e-08, 1.5848931924611136e-08, 1.7782794100389228e-08, 1.99526231496888e-08, 2.2387211385683398e-08, 2.51188643150958e-08, 2.8183829312644537e-08, 3.16227766016838e-08, 3.548133892335755e-08, 3.9810717055349736e-08, 4.466835921509632e-08, 5.0118723362727236e-08, 5.623413251903492e-08, 6.309573444801934e-08, 7.079457843841381e-08, 7.943282347242817e-08, 8.912509381337456e-08, 1.0000000000000001e-07, 1.1220184543019634e-07, 1.2589254117941672e-07, 1.4125375446227544e-07, 1.5848931924611136e-07, 1.778279410038923e-07, 1.9952623149688798e-07, 2.23872113856834e-07, 2.51188643150958e-07, 2.818382931264454e-07, 3.1622776601683797e-07, 3.548133892335755e-07, 3.9810717055349735e-07, 4.4668359215096317e-07, 5.011872336272724e-07, 5.623413251903491e-07, 6.309573444801933e-07, 7.07945784384138e-07, 7.943282347242816e-07, 8.912509381337455e-07, 1e-06, 1.1220184543019635e-06, 1.2589254117941674e-06, 1.4125375446227546e-06, 1.5848931924611137e-06, 1.7782794100389227e-06, 1.9952623149688796e-06, 2.23872113856834e-06, 2.51188643150958e-06, 2.818382931264454e-06, 3.1622776601683796e-06, 3.548133892335755e-06, 3.981071705534973e-06, 4.466835921509632e-06, 5.011872336272724e-06, 5.623413251903491e-06, 6.309573444801934e-06, 7.079457843841381e-06, 7.943282347242817e-06, 8.912509381337456e-06, 1e-05, 1.1220184543019633e-05, 1.2589254117941673e-05, 1.4125375446227545e-05, 1.5848931924611134e-05, 1.778279410038923e-05, 1.99526231496888e-05, 2.23872113856834e-05, 2.51188643150958e-05, 2.818382931264454e-05, 3.1622776601683795e-05, 3.5481338923357554e-05, 3.9810717055349735e-05, 4.466835921509632e-05, 5.011872336272724e-05, 5.6234132519034914e-05, 6.309573444801933e-05, 7.079457843841381e-05, 7.943282347242817e-05, 8.912509381337456e-05], "output array"=[15.8125, 35.625, 44.0625, 17.3125, 47.125, 32.875, 19.5, 12.625, 20.3125, 62.625, 53.75, 38.75, 45.75, 76.4375, 206.875, 198.5, 198.5625, 208.125, 217.4375, 206.875, 207.0, 175.625, 161.0, 154.125, 301.75, 313.75, 299.75, 298.1875, 441.125, 490.4375, 501.8125, 617.5, 619.4375, 629.6875, 780.5625, 917.1875, 931.5, 1056.8125, 1224.5, 1380.75, 1513.625, 1648.5, 1962.25, 2069.75, 2404.875, 2633.3125, 2979.375, 3271.5, 3737.375, 3908.375, 3950.875, 3963.5, 3980.25, 3991.125, 3999.1875, 4007.9375, 4009.875, 4010.0625, 4009.9375, 4010.0, 4010.0, 4010.0, 4009.9375, 4010.0, 4010.0, 4010.0, 4010.0625, 4009.875, 4010.0625, 4010.0, 4009.9375, 4009.9375, 4009.9375, 4009.8125, 4009.8125, 4009.9375, 4009.9375, 4010.0, 4009.9375, 4009.8125, 4010.0, 4009.8125, 4009.8125, 4009.9375, 4009.9375, 4009.75, 4009.75, 4009.875, 4009.875, 4009.8125, 4009.9375, 4009.9375, 4009.8125, 4009.75, 4009.875, 4010.0, 4009.9375, 4009.875, 4009.875, 4009.875, 4009.75, 4009.8125, 4009.8125, 4009.75, 4009.8125, 4009.75, 4009.8125, 4009.6875, 4009.6875, 4009.75, 4009.8125, 4009.75, 4009.75, 4009.6875, 4009.6875, 4009.625, 4009.625, 4009.6875, 4009.625, 4009.5625]}, {[1e-10, 1.1220184543019634e-10, 1.2589254117941675e-10, 1.4125375446227545e-10, 1.5848931924611137e-10, 1.778279410038923e-10, 1.9952623149688797e-10, 2.23872113856834e-10, 2.5118864315095804e-10, 2.8183829312644536e-10, 3.1622776601683795e-10, 3.5481338923357554e-10, 3.9810717055349735e-10, 4.466835921509632e-10, 5.011872336272724e-10, 5.623413251903491e-10, 6.309573444801933e-10, 7.07945784384138e-10, 7.943282347242817e-10, 8.912509381337457e-10, 1e-09, 1.1220184543019634e-09, 1.2589254117941673e-09, 1.4125375446227544e-09, 1.5848931924611136e-09, 1.7782794100389228e-09, 1.99526231496888e-09, 2.2387211385683402e-09, 2.5118864315095803e-09, 2.818382931264454e-09, 3.1622776601683795e-09, 3.548133892335755e-09, 3.981071705534974e-09, 4.466835921509632e-09, 5.011872336272724e-09, 5.623413251903492e-09, 6.309573444801934e-09, 7.079457843841381e-09, 7.943282347242815e-09, 8.912509381337456e-09, 1e-08, 1.1220184543019634e-08, 1.2589254117941673e-08, 1.4125375446227542e-08, 1.5848931924611136e-08, 1.7782794100389228e-08, 1.99526231496888e-08, 2.2387211385683398e-08, 2.51188643150958e-08, 2.8183829312644537e-08, 3.16227766016838e-08, 3.548133892335755e-08, 3.9810717055349736e-08, 4.466835921509632e-08, 5.0118723362727236e-08, 5.623413251903492e-08, 6.309573444801934e-08, 7.079457843841381e-08, 7.943282347242817e-08, 8.912509381337456e-08, 1.0000000000000001e-07, 1.1220184543019634e-07, 1.2589254117941672e-07, 1.4125375446227544e-07, 1.5848931924611136e-07, 1.778279410038923e-07, 1.9952623149688798e-07, 2.23872113856834e-07, 2.51188643150958e-07, 2.818382931264454e-07, 3.1622776601683797e-07, 3.548133892335755e-07, 3.9810717055349735e-07, 4.4668359215096317e-07, 5.011872336272724e-07, 5.623413251903491e-07, 6.309573444801933e-07, 7.07945784384138e-07, 7.943282347242816e-07, 8.912509381337455e-07, 1e-06, 1.1220184543019635e-06, 1.2589254117941674e-06, 1.4125375446227546e-06, 1.5848931924611137e-06, 1.7782794100389227e-06, 1.9952623149688796e-06, 2.23872113856834e-06, 2.51188643150958e-06, 2.818382931264454e-06, 3.1622776601683796e-06, 3.548133892335755e-06, 3.981071705534973e-06, 4.466835921509632e-06, 5.011872336272724e-06, 5.623413251903491e-06, 6.309573444801934e-06, 7.079457843841381e-06, 7.943282347242817e-06, 8.912509381337456e-06, 1e-05, 1.1220184543019633e-05, 1.2589254117941673e-05, 1.4125375446227545e-05, 1.5848931924611134e-05, 1.778279410038923e-05, 1.99526231496888e-05, 2.23872113856834e-05, 2.51188643150958e-05, 2.818382931264454e-05, 3.1622776601683795e-05, 3.5481338923357554e-05, 3.9810717055349735e-05, 4.466835921509632e-05, 5.011872336272724e-05, 5.6234132519034914e-05, 6.309573444801933e-05, 7.079457843841381e-05, 7.943282347242817e-05, 8.912509381337456e-05], "output array"=[6.0, 6.0625, 6.1875, 6.125, 6.125, 5.875, 5.8125, 5.5625, 6.0, 6.25, 6.125, 5.9375, 6.1875, 6.4375, 9.25, 8.9375, 8.25, 8.4375, 8.6875, 8.5625, 8.4375, 8.125, 7.9375, 7.75, 10.5625, 10.8125, 10.6875, 10.375, 12.625, 13.375, 13.5625, 15.3125, 15.25, 15.5, 17.875, 20.125, 20.0625, 22.75, 24.8125, 27.9375, 29.9375, 34.5625, 41.625, 44.625, 49.0, 53.625, 58.5, 64.5625, 71.875, 79.4375, 88.5, 96.9375, 112.625, 124.875, 133.75, 147.125, 168.1875, 187.6875, 208.0625, 236.8125, 259.6875, 288.4375, 326.375, 367.5625, 403.6875, 457.875, 512.6875, 571.875, 640.375, 718.0625, 802.625, 901.25, 1014.0625, 1135.1875, 1270.3125, 1418.75, 1591.875, 1787.8125, 2000.625, 2242.3125, 2513.625, 2816.8125, 3157.6875, 3544.25, 3876.875, 3932.25, 3955.5625, 3970.6875, 3982.125, 3992.0, 4000.375, 4006.3125, 4006.3125, 4006.375, 4006.3125, 4006.3125, 4006.3125, 4006.3125, 4006.3125, 4006.3125, 4006.3125, 4006.3125, 4006.3125, 4006.25, 4006.3125, 4006.375, 4006.3125, 4006.375, 4006.3125, 4006.25, 4006.3125, 4006.375, 4006.375, 4006.375, 4006.375, 4006.375, 4006.3125, 4006.375, 4006.375, 4006.4375]}, {[1e-10, 1.1220184543019634e-10, 1.2589254117941675e-10, 1.4125375446227545e-10, 1.5848931924611137e-10, 1.778279410038923e-10, 1.9952623149688797e-10, 2.23872113856834e-10, 2.5118864315095804e-10, 2.8183829312644536e-10, 3.1622776601683795e-10, 3.5481338923357554e-10, 3.9810717055349735e-10, 4.466835921509632e-10, 5.011872336272724e-10, 5.623413251903491e-10, 6.309573444801933e-10, 7.07945784384138e-10, 7.943282347242817e-10, 8.912509381337457e-10, 1e-09, 1.1220184543019634e-09, 1.2589254117941673e-09, 1.4125375446227544e-09, 1.5848931924611136e-09, 1.7782794100389228e-09, 1.99526231496888e-09, 2.2387211385683402e-09, 2.5118864315095803e-09, 2.818382931264454e-09, 3.1622776601683795e-09, 3.548133892335755e-09, 3.981071705534974e-09, 4.466835921509632e-09, 5.011872336272724e-09, 5.623413251903492e-09, 6.309573444801934e-09, 7.079457843841381e-09, 7.943282347242815e-09, 8.912509381337456e-09, 1e-08, 1.1220184543019634e-08, 1.2589254117941673e-08, 1.4125375446227542e-08, 1.5848931924611136e-08, 1.7782794100389228e-08, 1.99526231496888e-08, 2.2387211385683398e-08, 2.51188643150958e-08, 2.8183829312644537e-08, 3.16227766016838e-08, 3.548133892335755e-08, 3.9810717055349736e-08, 4.466835921509632e-08, 5.0118723362727236e-08, 5.623413251903492e-08, 6.309573444801934e-08, 7.079457843841381e-08, 7.943282347242817e-08, 8.912509381337456e-08, 1.0000000000000001e-07, 1.1220184543019634e-07, 1.2589254117941672e-07, 1.4125375446227544e-07, 1.5848931924611136e-07, 1.778279410038923e-07, 1.9952623149688798e-07, 2.23872113856834e-07, 2.51188643150958e-07, 2.818382931264454e-07, 3.1622776601683797e-07, 3.548133892335755e-07, 3.9810717055349735e-07, 4.4668359215096317e-07, 5.011872336272724e-07, 5.623413251903491e-07, 6.309573444801933e-07, 7.07945784384138e-07, 7.943282347242816e-07, 8.912509381337455e-07, 1e-06, 1.1220184543019635e-06, 1.2589254117941674e-06, 1.4125375446227546e-06, 1.5848931924611137e-06, 1.7782794100389227e-06, 1.9952623149688796e-06, 2.23872113856834e-06, 2.51188643150958e-06, 2.818382931264454e-06, 3.1622776601683796e-06, 3.548133892335755e-06, 3.981071705534973e-06, 4.466835921509632e-06, 5.011872336272724e-06, 5.623413251903491e-06, 6.309573444801934e-06, 7.079457843841381e-06, 7.943282347242817e-06, 8.912509381337456e-06, 1e-05, 1.1220184543019633e-05, 1.2589254117941673e-05, 1.4125375446227545e-05, 1.5848931924611134e-05, 1.778279410038923e-05, 1.99526231496888e-05, 2.23872113856834e-05, 2.51188643150958e-05, 2.818382931264454e-05, 3.1622776601683795e-05, 3.5481338923357554e-05, 3.9810717055349735e-05, 4.466835921509632e-05, 5.011872336272724e-05, 5.6234132519034914e-05, 6.309573444801933e-05, 7.079457843841381e-05, 7.943282347242817e-05, 8.912509381337456e-05], "output array"=[7.25, 7.1875, 7.1875, 7.25, 7.25, 7.1875, 7.3125, 7.25, 7.1875, 7.25, 7.25, 7.1875, 7.25, 7.25, 7.3125, 7.25, 7.25, 7.3125, 7.3125, 7.3125, 7.375, 7.3125, 7.3125, 7.25, 7.375, 7.4375, 7.3125, 7.4375, 7.375, 7.5, 7.5, 7.625, 7.5625, 7.5, 7.5625, 7.75, 7.6875, 7.8125, 7.8125, 7.875, 8.0625, 8.125, 8.25, 8.3125, 8.4375, 8.6875, 8.8125, 8.9375, 9.25, 9.375, 9.8125, 10.0, 10.25, 10.6875, 11.1875, 11.625, 12.1875, 12.875, 13.5625, 14.3125, 15.125, 16.125, 17.125, 18.25, 19.5, 21.1875, 22.875, 24.8125, 26.9375, 29.8125, 34.125, 39.375, 43.8125, 47.6875, 52.0, 56.8125, 62.625, 69.3125, 76.375, 83.8125, 92.6875, 107.0, 118.25, 128.75, 140.5, 155.6875, 177.8125, 198.0, 219.625, 248.8125, 272.8125, 308.25, 343.3125, 385.0, 431.1875, 481.875, 534.375, 601.1875, 671.5625, 758.5, 847.125, 949.8125, 1062.1875, 1190.75, 1334.4375, 1494.75, 1672.4375, 1877.3125, 2102.375, 2358.0, 2641.8125, 2960.6875, 3322.5, 3719.875, 3911.125, 3946.3125, 3965.4375, 3979.0, 3990.25, 3999.8125]}]
  in  "ISweep 2":bool
  in  "milliseconds stabilisation 2":u32=10
  in  "SWIR/MWIR 2":bool=TRUE
  in  "SuperAvg":i32=1 min=1 max=100
  in  "Other Channel Forcing":dbl min=0.0 max=10.0 format="%#_13g"
  in  "DAC":i32 min=0 max=4095 step=1
  in  "Modulation Steps":i32=2 min=2 max=1000 step=1
  in  "Modulation Max":dbl min=0.0 max=10.0
  in  "Modulation Min":dbl min=-10.0 max=10.0
  in  "SweepLight":bool
  in  "Detector 7":u16(ring) items=["SWIR", "MWIR"]
  out "Output vs Light":cluster{dbl[], dbl[]}[](graph)
  in  "Gain 2":u16(ring) items=["High", "Med", "Low"]
  in  "Abort 2":bool
  in  "SweepVDAC":bool
  in  "ISource":dbl min=-1e-06 max=1e-06
  in  "VDAC Step":i32=1 min=1 max=100
  in  "VDAC Max":i32 min=0 max=4095
  in  "VDAC Min":i32 min=0 max=4000
  in  "Detector 5":u16(ring) items=["SWIR", "MWIR"]
  out "VDAC Sweep":cluster{dbl[], dbl[]}[](graph)
  in  "Abort SweepVDAC":bool
  in  "Channel":u16(ring) items=["SWIR - High", "SWIR - Med", "SWIR - Low", "MWIR - High", "MWIR - Med", "MWIR - Low", "TRP 1", "TRP 2"]
  out "XY Graph":cluster{"output array":dbl[], dbl[]}(graph)
  in  "NoiseSweep":bool
  in  "SamplesToAverage":i32=100
  out "exit":bool
  # "3.3V supply"
  # "Heater"
  # "+12V Supply"
  # "-12V Supply"
  # "Pause button will halt collection and display.\nThis allows graph to be printed etc."
  # "Burst mode is intended to examine behaviour of the ADC\n\nA burst of readings is recorded on the EGSE and then gathered here."
  # "Light source modulated by USB205L working as voltage source connected to MOD input of LD250C\nreference photodiode monitored by 6846 picoammeter"
  # "Measure PSU noise immmunity by applying different frequencies via TG5011A and recording pk-pk noise on SWIR High gain channel over 1000 measurements\nFrequencies from 1Hz - 1KHz at 20 points/decade"
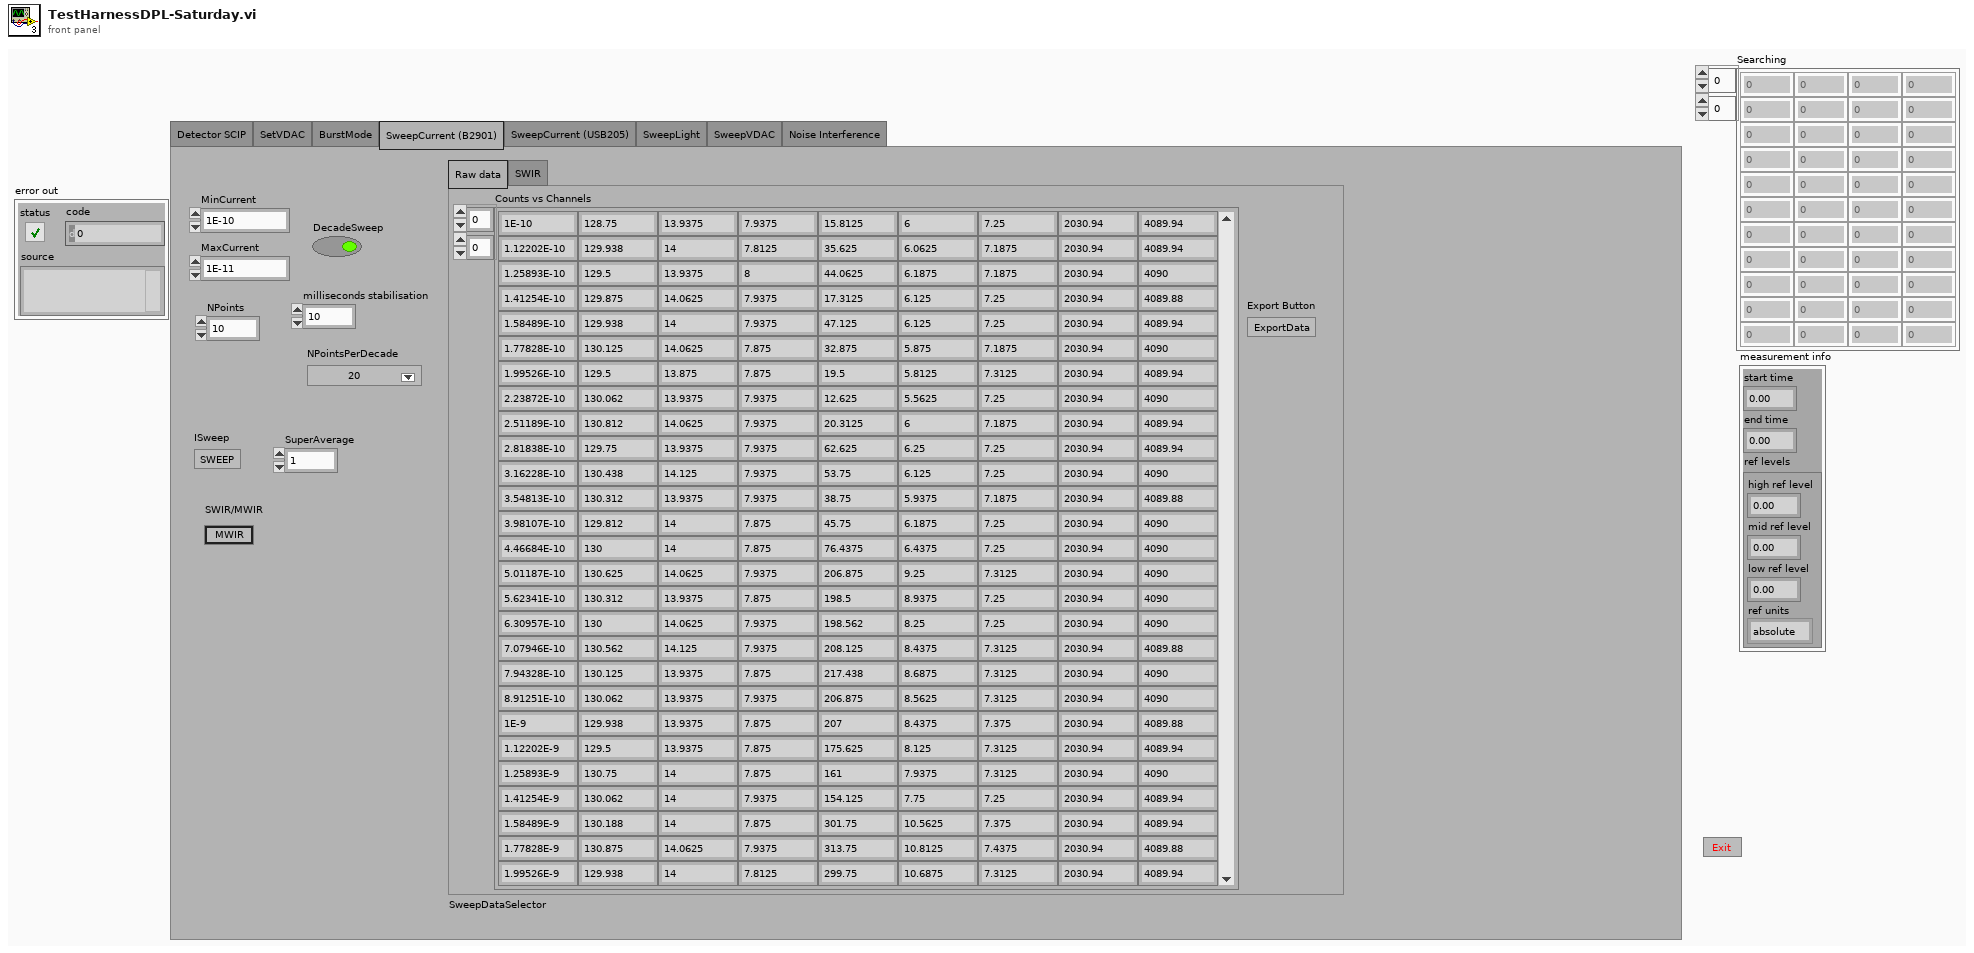
[diagram p1: front panel]
types:
  T1 = cluster{"start time":dbl, "end time":dbl, "ref levels":cluster{"high ref level":dbl, "mid ref level":dbl, "low ref level":dbl, "ref units":u16}}
  T2 = enum32{"Detector SCIP", "SetVDAC", "BurstMode", "SweepCurrent (B2901)", "SweepCurrent (USB205)", "SweepLight", "SweepVDAC", "Noise Interference"}
  T3 = cluster{"Name":string, "DAC Offset":i32, "DAC StepsPerHGCount":dbl}[]
  T4 = cluster{"subarray[0]":dbl, "subarray[1]":dbl, "subarray[2]":dbl, "subarray[3]":dbl, "subarray[4]":dbl, "subarray[5]":dbl, "subarray[6]":dbl, "subarray[7]":dbl, "subarray[8]":dbl}
  T5 = cluster{"Baud Rate":u32, "Parity":u16, "Data Bits":u16, "Stop Bits":u16, "Flow Control":u16}
  T6 = cluster{"high ref level":dbl, "mid ref level":dbl, "low ref level":dbl, "ref units":u16}
  T7 = cluster{"ScienceData[0]":dbl, "ScienceData[1]":dbl, "ScienceData[2]":dbl, "ScienceData[3]":dbl, "ScienceData[4]":dbl, "ScienceData[5]":dbl, "ScienceData[6]":dbl, "ScienceData[7]":dbl, "ScienceData[8]":dbl}
  T8 = cluster{"method":enum32{"histogram", "peak", "auto select"}, "histogram size":i32, "histogram method":enum16{"mode"}, "reserved":dbl}
  T9 = cluster{"Name":string, "DAC Offset":i32, "DAC StepsPerHGCount":dbl}
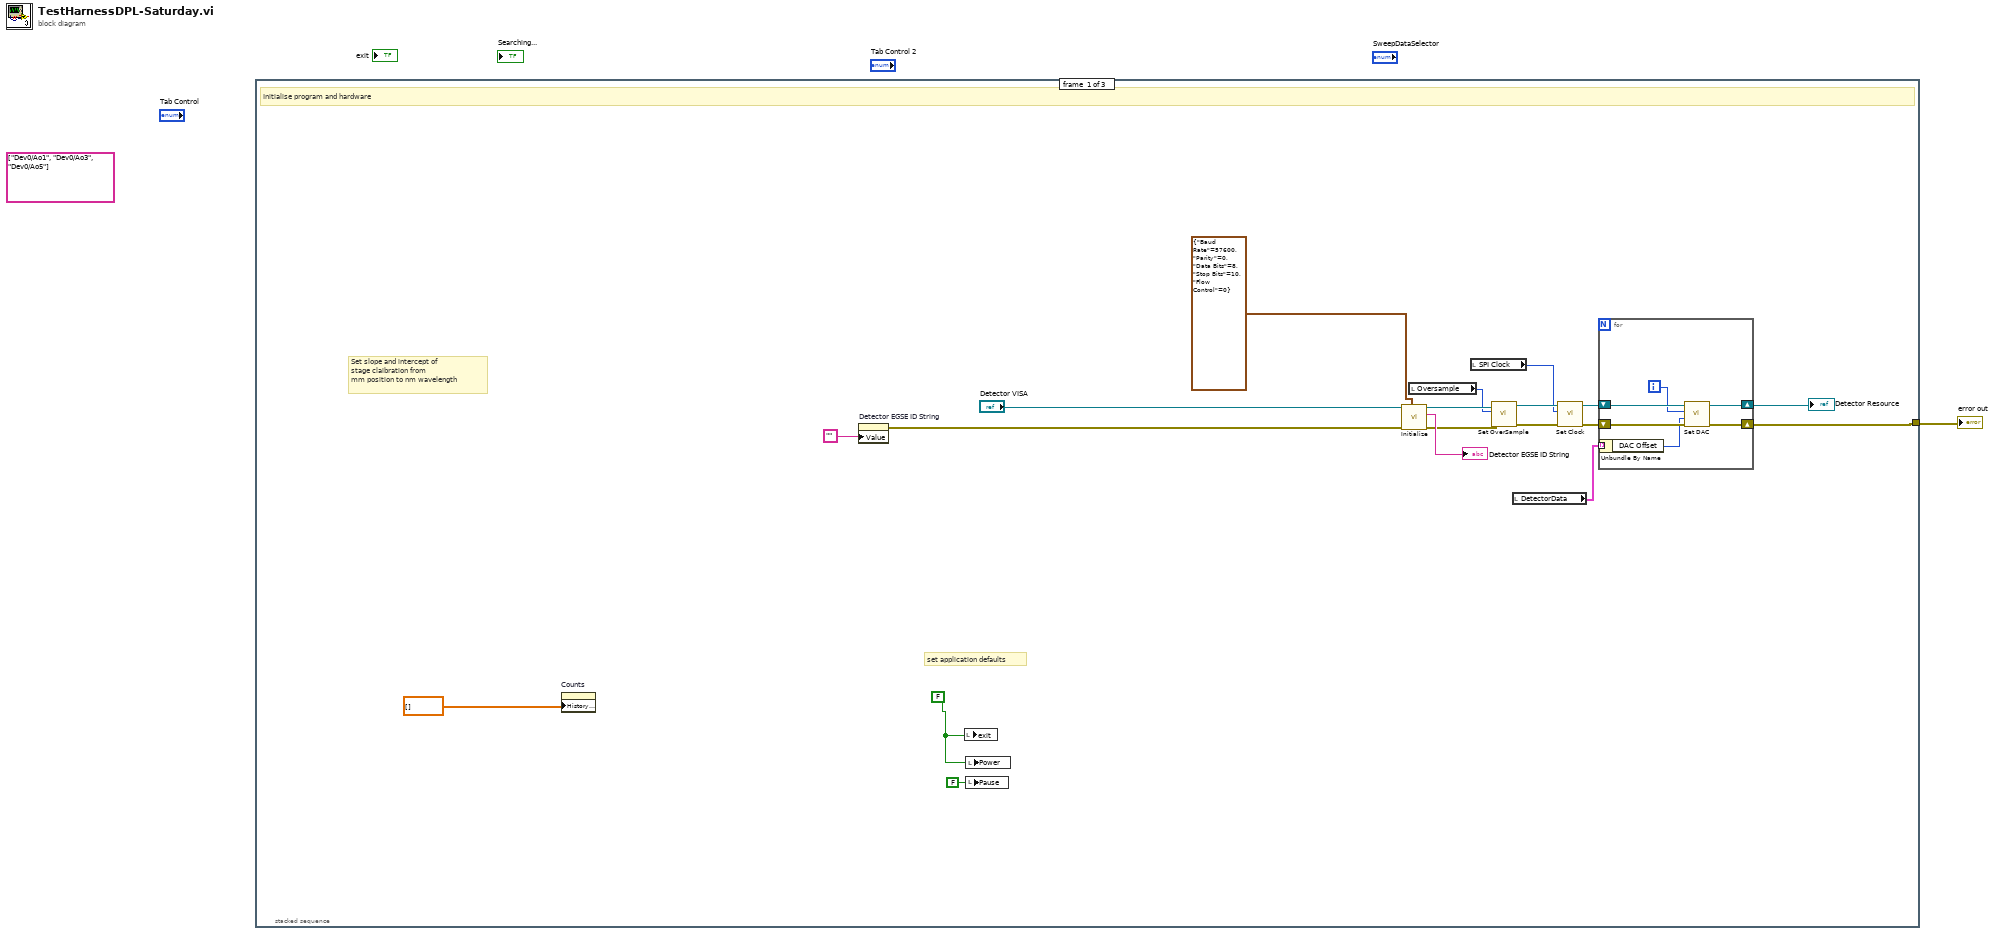
[diagram p0: block diagram]
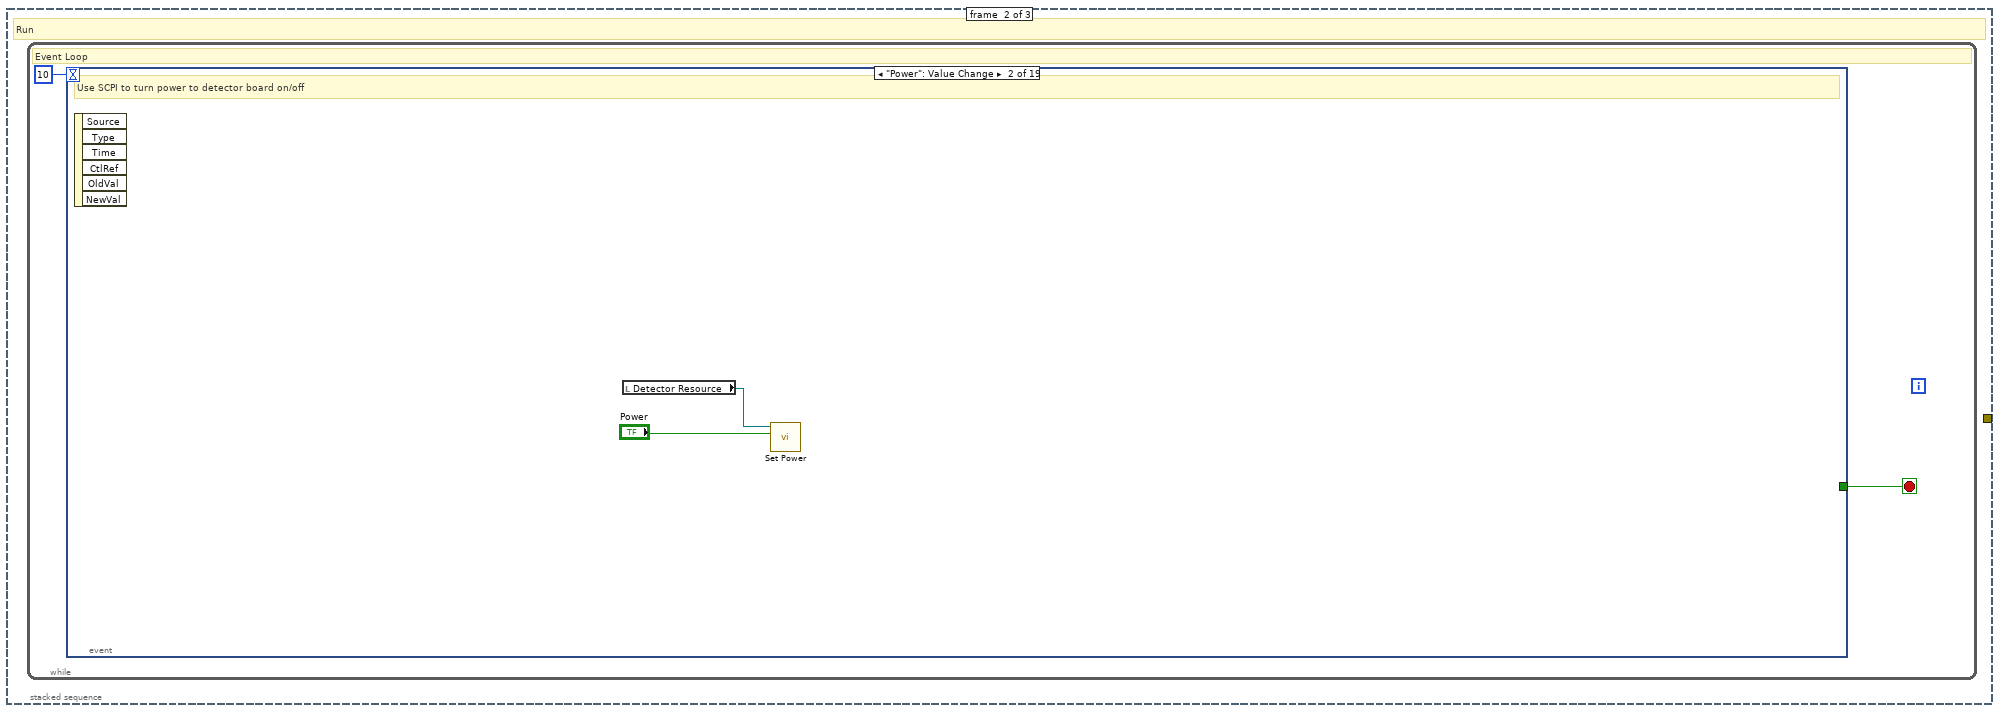
[diagram p2: hidden frame]
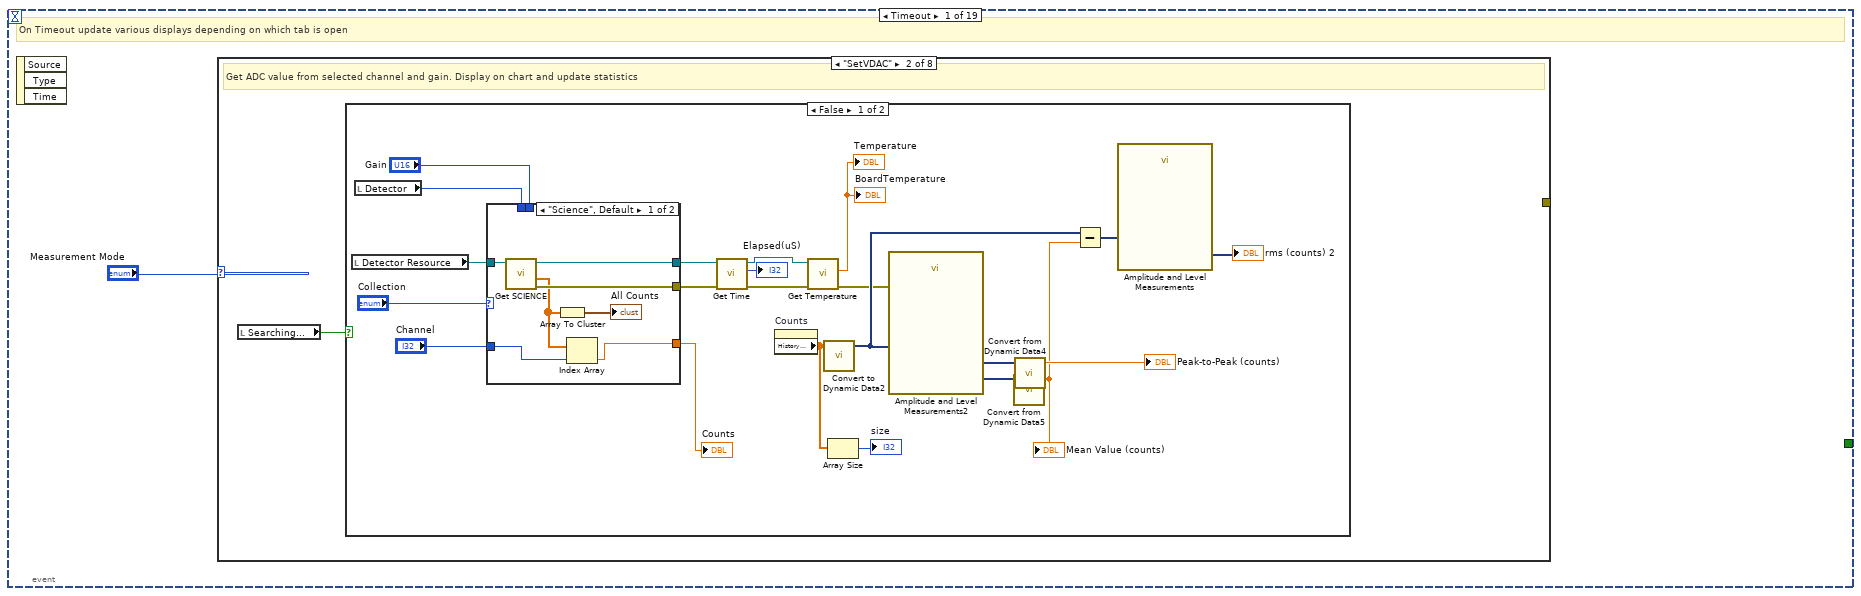
[diagram p3: hidden frame]
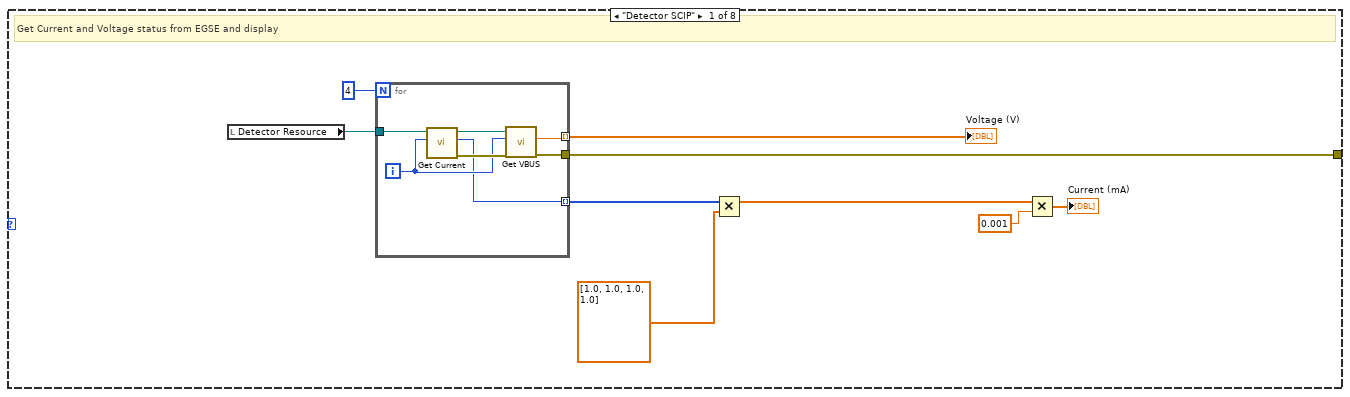
[diagram p4: hidden frame]
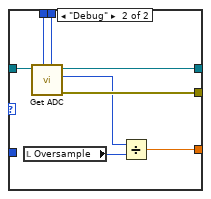
[diagram p5: hidden frame]
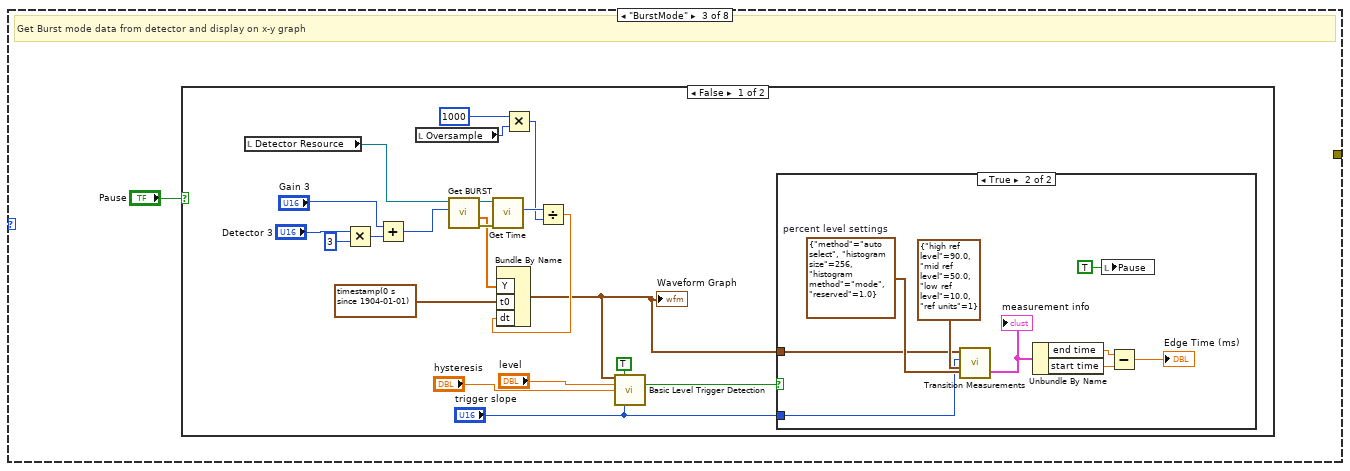
[diagram p7: hidden frame]
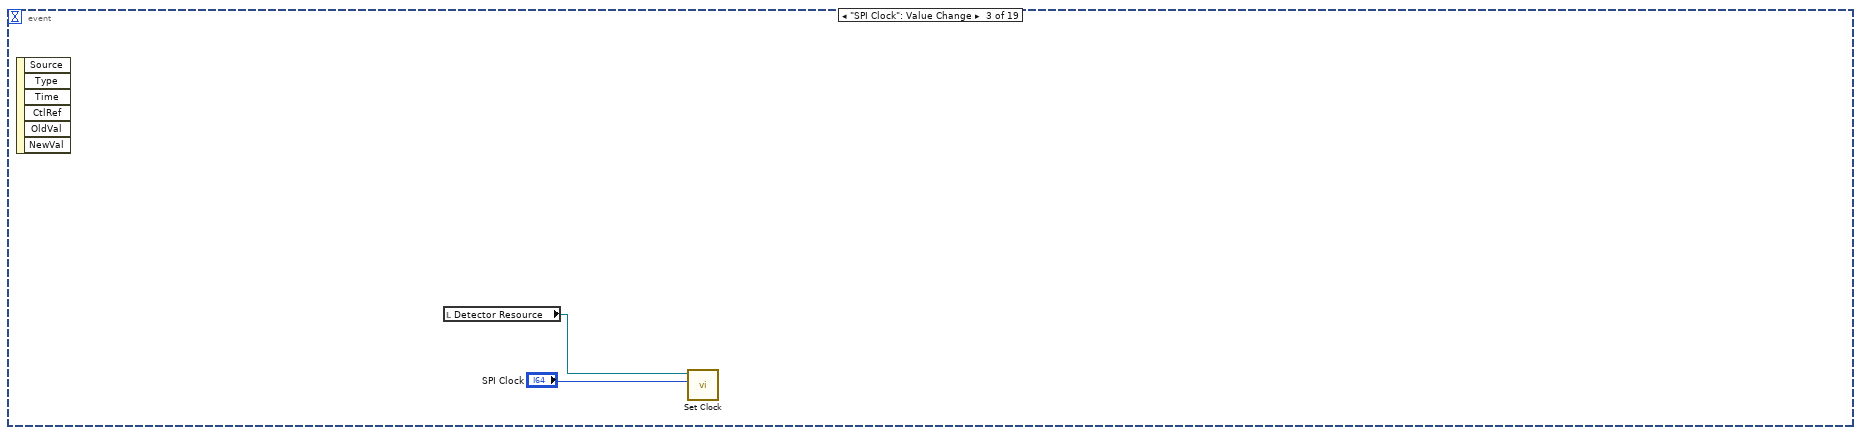
[diagram p15: hidden frame]
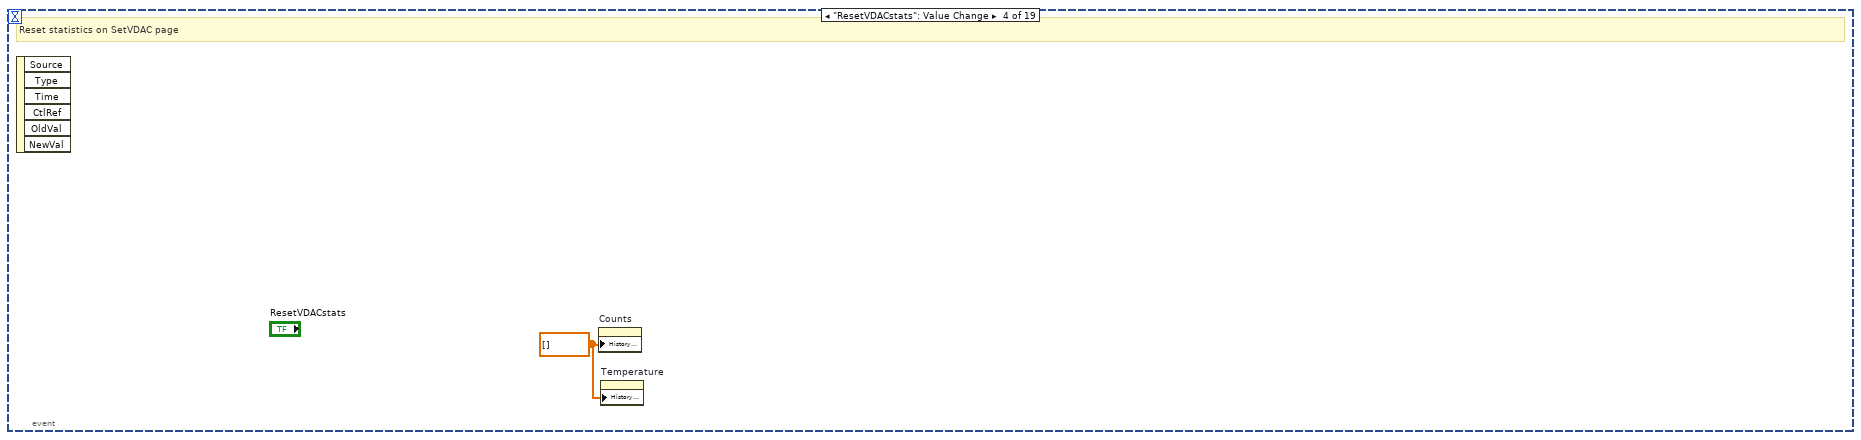
[diagram p16: hidden frame]
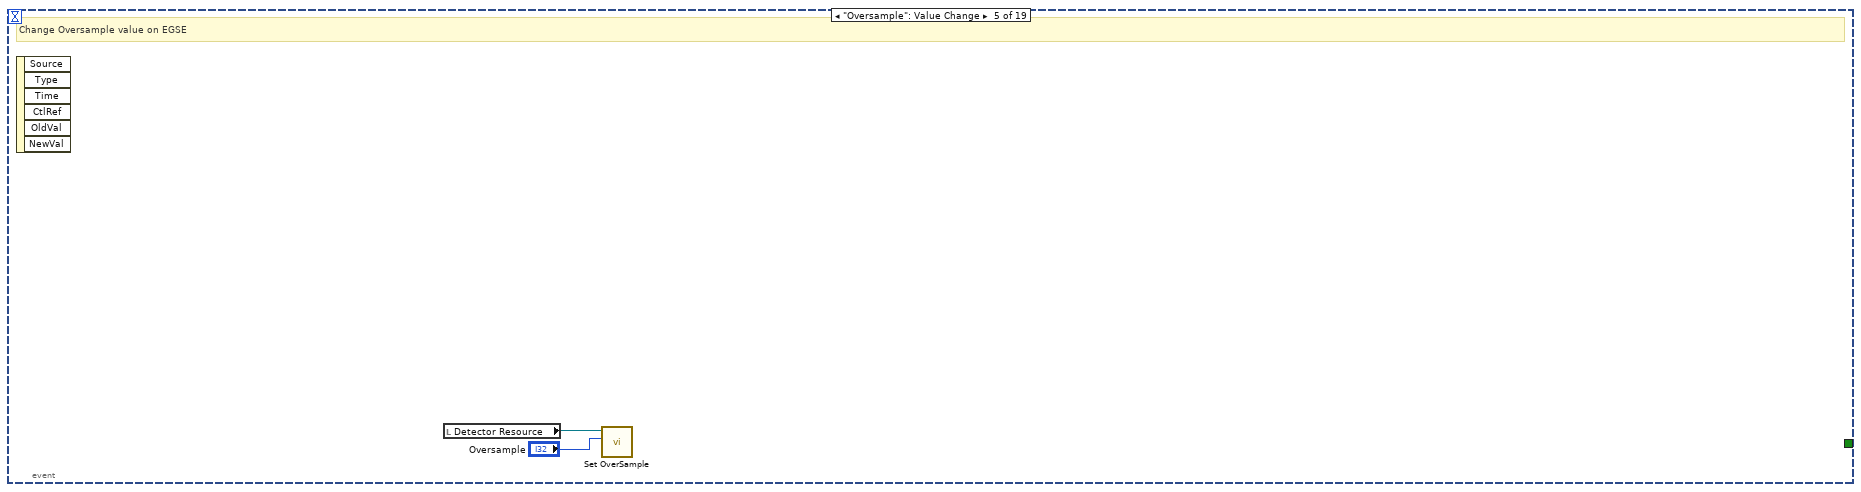
[diagram p17: hidden frame]
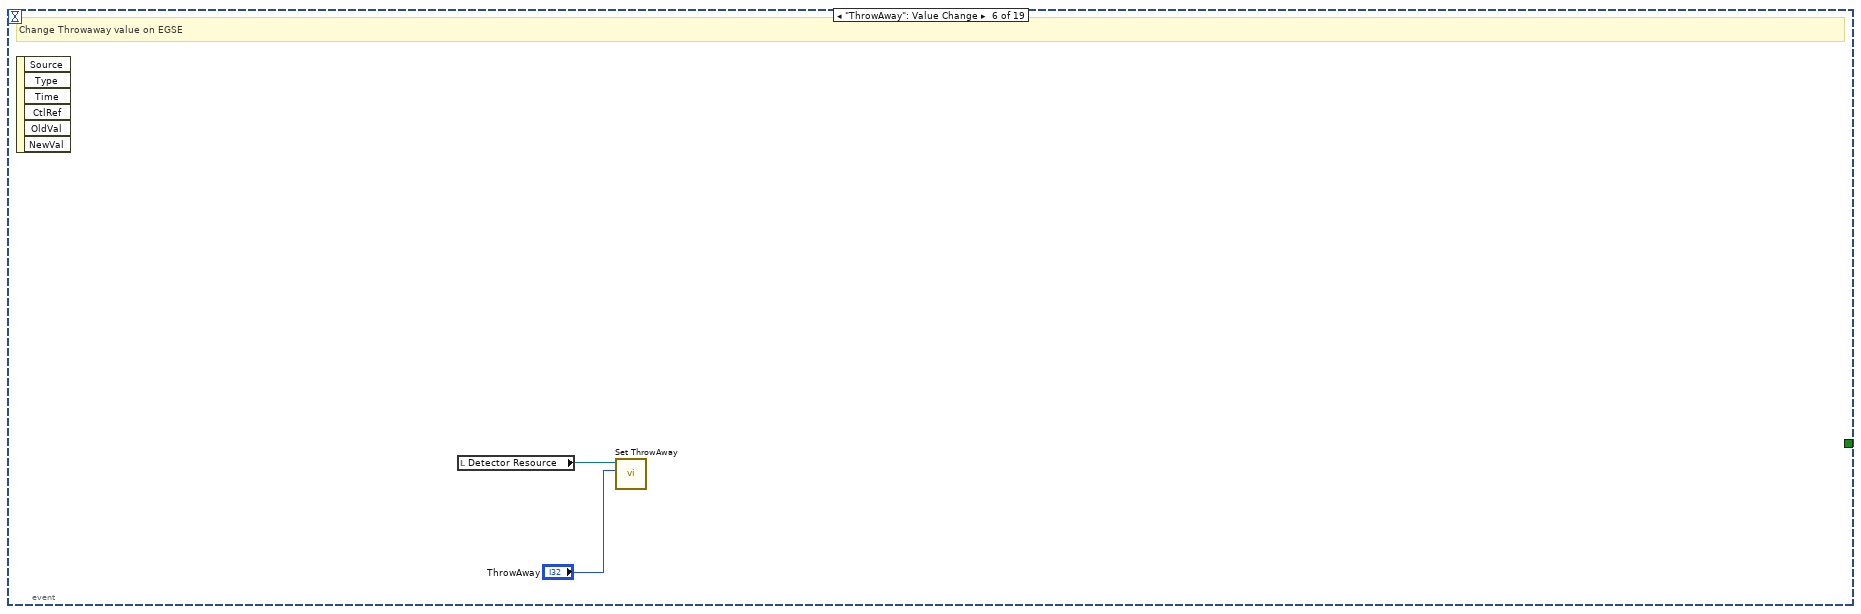
[diagram p18: hidden frame]
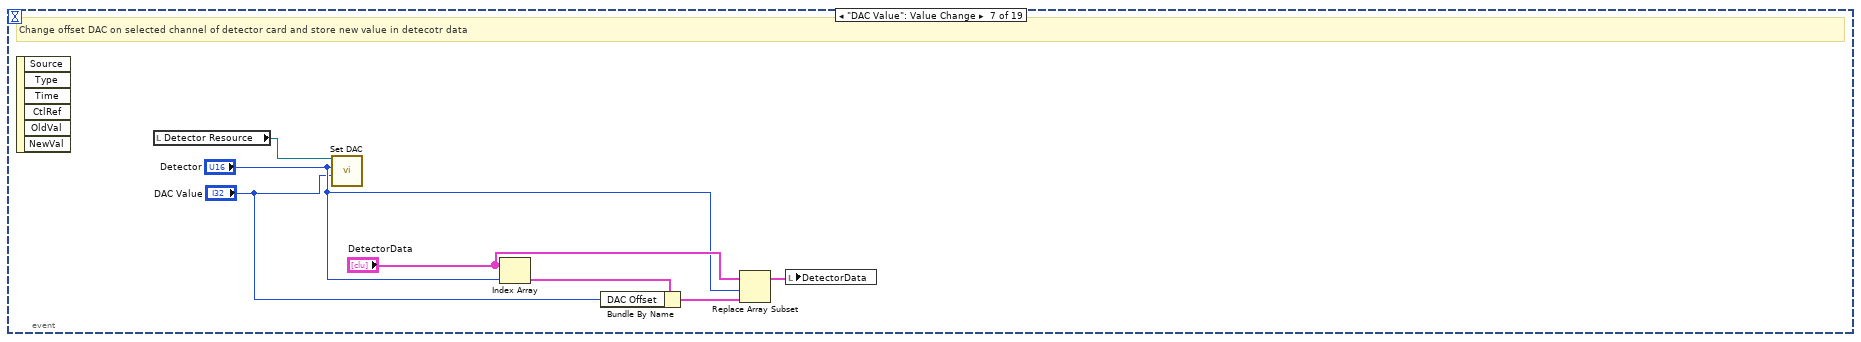
[diagram p19: hidden frame]
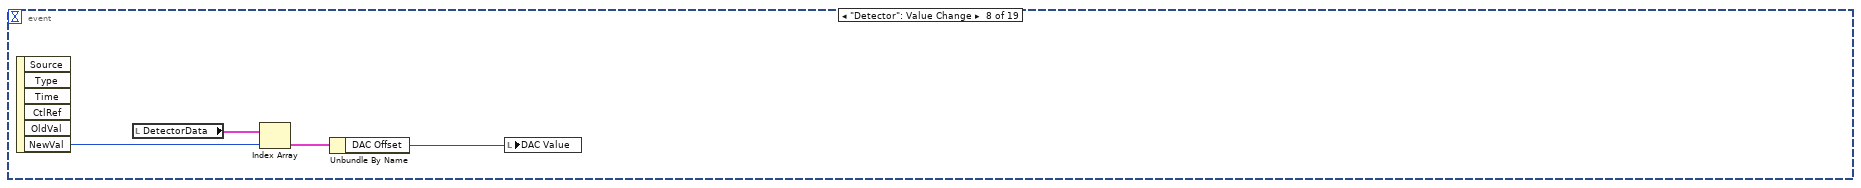
[diagram p20: hidden frame]
diagram:
  (unwired) string[] ["Dev0/Ao1", "Dev0/Ao3", "Dev0/Ao5"]
  n1 = stacked-sequence {
    tunnel: [w3 _ _] -> w1
    frame #0 {
      w19 = FALSE ("connected")
      # "Set slope and intercept of \nstage claibration from\nmm position to nm wavelength"
      # "set application defaults"
      # "Initialise program and hardware"
      n2 = property on="Counts" class="WFChart (strict)"("History Data"=dbl[] []) -> ()  [unwired: 2 in, 2 out]
      n3 = property on="Detector EGSE ID String" class="Str"("Value"="") -> (error out=w17:errorcluster)  [unwired: 2 in, 1 out]
      n4 = local write "exit"(w19) -> ()
      n5 = local write "Power"(w19) -> ()
      n6 = local write "Pause"(FALSE ("Pause")) -> ()
      n7 = call <instrlib>:"Initialize.vi"("Serial Configuration"=T5 {"Baud Rate"=57600, "Parity"=0, "Data Bits"=8, "Stop Bits"=10, "Flow Control"=0}, "error in (no error)"=w17, "VISA resource name"="Detector VISA") -> ("error out"=w13:errorcluster, "ID String"=→"Detector EGSE ID String":string, "VISA resource name out"=w12:refnum<visa-resource-name>)  [unwired: 6 in]
      n8 = local read "Oversample"() -> (w11:i32)
      n9 = local read "SPI Clock"() -> (w6:i64)
      n10 = call <instrlib>:"Set OverSample.vi"("error in (no error)"=w13, "oversample (0)"=w11, "VISA resource name"=w12) -> ("error out"=w10:errorcluster, "VISA resource name out"=w8:refnum<visa-resource-name>)  [unwired: 7 in]
      n11 = local read "DetectorData"() -> (w2:T3)
      n12 = call <instrlib>:"Set Clock.vi"("error in (no error)"=w10, "ClockSpeed"=w6, "VISA resource name"=w8) -> ("error out"=w9:errorcluster, "VISA resource name out"=w7:refnum<visa-resource-name>)  [unwired: 7 in]
      n13 = for {
        shift-right: [w24] -> w3
        shift-left: w9 -> [w26]
        shift-right: [w27] -> w14
        shift-left: w7 -> [w25]
        tunnel: w2 -> [w23] mode=indexing
        i -> [w22]
        n14 = Unbundle By Name(w23) -> ("DAC Offset"=w21:i32)
        n15 = call <instrlib>:"Set DAC.vi"("error in (no error)"=w26, "value (0)"=w21, "chan (0)"=w22, "VISA resource name"=w25) -> ("error out"=w24:errorcluster, "VISA resource name out"=w27:refnum<visa-resource-name>)  [unwired: 6 in]
      }
      "Detector Resource" <- w14
    }
    frame #1 {
      # "Run"
      n16 = while {
        stop <- w28 stop-if-true
        # "Event Loop"
        n17 = event shown="[1] \"Power\": Value Change" {
          selector: _ -> [_ _ _ _ _ _ _ _ _ _ _ _ _ _ _ _ _ _ _]
          dyn-events: _ -> [_ _ _ _ _ _ _ _ _ _ _ _ _ _ _ _ _ _ _]
          timeout: 10 -> [_ _ _ _ _ _ _ _ _ _ _ _ _ _ _ _ _ _ _]
          tunnel: [_ _ _ _ _ _ _ _ _ _ _ _ _ _ _ _ _ "Exit" _] -> w28
          event Timeout {
            # "On Timeout update various displays depending on which tab is open"
            n18 = event-data() -> ()  [unwired: 1 in, 3 out]
            n19 = case shown="\"SetVDAC\"" "Measurement Mode" {
              tunnel: [w31 _ _ _ _ _ _ _] -> _
              frame "Detector SCIP" {
                # "Get Current and Voltage status from EGSE and display"
                n20 = local read "Detector Resource"() -> (w39:refnum<visa-resource-name>)
                n21 = for {
                  N: 4 -> [_]
                  tunnel: w39 -> [w46]
                  tunnel: [w42] -> w36 mode=indexing
                  tunnel: [w41] -> w37 mode=indexing
                  tunnel: [w40] -> w31
                  i -> [w43]
                  n22 = call <instrlib>:"Get Current.vi"("chan (1)"=w43, "VISA resource name"=w46) -> ("error out"=w45:errorcluster, "output"=w42:i32, "VISA resource name out"=w44:refnum<visa-resource-name>)  [unwired: 7 in]
                  n23 = call <instrlib>:"Get VBUS.vi"("error in (no error)"=w45, "chan (1)"=w43, "VISA resource name"=w44) -> ("error out"=w40:errorcluster, "output"=w41:dbl)  [unwired: 6 in, 1 out]
                }
                "Voltage (V)" <- w37
                n24 = Multiply(x=w36, y=dbl[] [1.0, 1.0, 1.0, 1.0]) -> (x*y=w33:dbl[])
                n25 = Multiply(x=w33, y=0.001) -> (x*y=→"Current (mA)":dbl[])
              }
              frame "SetVDAC" {
                # "Get ADC value from selected channel and gain. Display on chart and update statistics"
                n26 = local read "Searching..."() -> (w47:bool)
                n27 = case shown="False" w47 {
                  frame False {
                    n28 = local read "Detector Resource"() -> (w69:refnum<visa-resource-name>)
                    n29 = local read "Detector"() -> (w67:u16)
                    n30 = case shown="\"Science\", Default" "Collection" {
                      tunnel: w69 -> [w76 w84]
                      tunnel: "Gain" -> [_ w83]
                      tunnel: w67 -> [_ w82]
                      tunnel: [w75 w81] -> w66
                      tunnel: [w74 w80] -> w65
                      tunnel: [w72 w78] -> w49
                      tunnel: "Channel" -> [w73 _]
                      frame "Science", Default {
                        n31 = call <instrlib>:"Get SCIENCE.vi"("VISA resource name"=w76) -> ("error out"=w74:errorcluster, "ScienceData"=w71:dbl[], "VISA resource name out"=w75:refnum<visa-resource-name>)  [unwired: 7 in, 1 out]
                        n32 = Array To Cluster(array=w71) -> (cluster=→"All Counts":T7)
                        n33 = Index Array(array=w71, index=w73) -> (element=w72:dbl)
                      }
                      frame "Debug" {
                        n34 = local read "Oversample"() -> (w79:i32)
                        n35 = call <instrlib>:"Get ADC.vi"("Gain"=w83, "Detector"=w82, "VISA resource name"=w84) -> ("error out"=w80:errorcluster, "output"=w77:i32, "VISA resource name out"=w81:refnum<visa-resource-name>)  [unwired: 6 in]
                        n36 = Divide(x=w77, y=w79) -> (x/y=w78:dbl)
                      }
                    }
                    "Counts" <- w49
                    n37 = call <instrlib>:"Get Time.vi"("error in (no error)"=w65, "VISA resource name"=w66) -> ("error out"=w53:errorcluster, "output"=→"Elapsed(uS)":i32, "VISA resource name out"=w51:refnum<visa-resource-name>)  [unwired: 7 in]
                    n38 = property on="Counts" class="WFChart (strict)"() -> ("History Data"=w56:dbl[])  [unwired: 2 in, 2 out]
                    n39 = call <instrlib>:"Get Temperature.vi"("error in (no error)"=w53, "VISA resource name"=w51) -> ("error out"=w52:errorcluster, "output"=→"Temperature" →"BoardTemperature":dbl)  [unwired: 7 in, 1 out]
                    n40 = call "Convert to Dynamic Data2"("Array"=w56) -> ("Dynamic Data Type"=w57:dynamicdata)  [unwired: 3 in]
                    n41 = Array Size(array=w56) -> (size(s)=→"size":i32)
                    n42 = call "Amplitude and Level Measurements2"("Signals"=w57, "error in (no error)"=w52) -> ("Mean (DC)"=w59:dynamicdata, "Peak to Peak"=w62:dynamicdata)  [unwired: 10 in, 2 out]
                    n43 = call "Convert from Dynamic Data5"("Dynamic Data Type"=w59) -> ("Scalar"=w58:dbl)  [unwired: 3 in]
                    "Mean Value (counts)" <- w58
                    n44 = call "Convert from Dynamic Data4"("Dynamic Data Type"=w62) -> ("Scalar"=→"Peak-to-Peak (counts)":dbl)  [unwired: 3 in]
                    n45 = Subtract(x=w57, y=w58) -> (x-y=w60:dynamicdata)
                    n46 = call "Amplitude and Level Measurements"("Signals"=w60) -> ("RMS"=→"rms (counts) 2":dynamicdata)  [unwired: 11 in, 3 out]
                  }
                  frame True {
                  }
                }
              }
              frame "BurstMode" {
                # "Get Burst mode data from detector and display on x-y graph"
                n47 = case shown="False" "Pause" {
                  frame False {
                    n48 = local read "Detector Resource"() -> (w106:refnum<visa-resource-name>)
                    n49 = Multiply(x="Detector 3", y=u16 3) -> (x*y=w105:u16)
                    n50 = Add(x="Gain 3", y=w105) -> (x+y=w103:u16)
                    n51 = local read "Oversample"() -> (w98:i32)
                    n52 = call <instrlib>:"Get BURST.vi"("chan (0)"=w103, "VISA resource name"=w106) -> ("error out"=w100:errorcluster, "subarray"=w94:dbl[], "VISA resource name out"=w99:refnum<visa-resource-name>)  [unwired: 6 in, 1 out]
                    n53 = call <instrlib>:"Get Time.vi"("error in (no error)"=w100, "VISA resource name"=w99) -> ("output"=w97:i32)  [unwired: 7 in, 2 out]
                    n54 = Multiply(x=1000, y=w98) -> (x*y=w96:i32)
                    n55 = Divide(x=w97, y=w96) -> (x/y=w93:dbl)
                    n56 = Bundle By Name("Y"=w94, "t0"=timestamp(0 s since 1904-01-01), "dt"=w93) -> (w86:waveform(dbl))  [unwired: 1 in]
                    "Waveform Graph" <- w86
                    n57 = call-poly <vilib>:"Basic Level Trigger Detection.vi"("signal in"=w86, "reset"=TRUE, "level"="level", "hysteresis"="hysteresis", "trigger slope"="trigger slope") -> ("trigger detected?"=w90:bool)  [unwired: 8 in, 2 out]
                    n58 = case shown="True" w90 {
                      tunnel: w86 -> [_ w112]
                      tunnel: "trigger slope" -> [_ w111]
                      frame False {
                      }
                      frame True {
                        w114 = T8 {"method"=enum."auto select", "histogram size"=256, "histogram method"=enum."mode", "reserved"=1.0}  # percent level settings
                        n59 = call-poly <vilib>:"Transition Measurements.vi"("percent level settings"=w114, "reference levels"=T6 {"high ref level"=90.0, "mid ref level"=50.0, "low ref level"=10.0, "ref units"=1}, "polarity (rising)"=w111, "signal in"=w112) -> ("measurement info"=w110:T1)  [unwired: 2 in, 5 out]
                        "measurement info" <- w110
                        n60 = Unbundle By Name(w110) -> ("end time"=w108:dbl, "start time"=w109:dbl)
                        n61 = local write "Pause"(TRUE ("Pause")) -> ()
                        n62 = Subtract(x=w108, y=w109) -> (x-y=→"Edge Time (ms)":dbl)
                      }
                    }
                  }
                  frame True {
                  }
                }
              }
              frame "SweepCurrent (B2901)" {
              }
              frame "SweepVDAC" {
              }
              frame "Noise Interference" {
              }
              frame "SweepLight" {
              }
              frame "SweepCurrent (USB205)" {
              }
            }
          }
          event "Power": Value Change {
            # "Use SCPI to turn power to detector board on/off"
            n63 = event-data() -> ()  [unwired: 1 in, 6 out]
            n64 = local read "Detector Resource"() -> (w117:refnum<visa-resource-name>)
            n65 = call <instrlib>:"Set Power.vi"("Power (0)"="Power", "VISA resource name"=w117) -> ()  [unwired: 8 in, 2 out]
          }
          event "SPI Clock": Value Change {
            n66 = event-data() -> ()  [unwired: 1 in, 6 out]
            n67 = local read "Detector Resource"() -> (w119:refnum<visa-resource-name>)
            n68 = call <instrlib>:"Set Clock.vi"("ClockSpeed"="SPI Clock", "VISA resource name"=w119) -> ()  [unwired: 8 in, 2 out]
          }
          event "ResetVDACstats": Value Change {
            w120 = dbl[] [] ("History Data")
            # "Reset statistics on SetVDAC page"
            n69 = event-data() -> ()  [unwired: 1 in, 6 out]
            n70 = property on="Counts" class="WFChart (strict)"("History Data"=w120) -> ()  [unwired: 2 in, 2 out]
            n71 = property on="Temperature" class="WFChart (strict)"("History Data"=w120) -> ()  [unwired: 2 in, 2 out]
          }
          event "Oversample": Value Change {
            # "Change Oversample value on EGSE"
            n72 = event-data() -> ()  [unwired: 1 in, 6 out]
            n73 = local read "Detector Resource"() -> (w122:refnum<visa-resource-name>)
            n74 = call <instrlib>:"Set OverSample.vi"("oversample (0)"="Oversample", "VISA resource name"=w122) -> ()  [unwired: 8 in, 2 out]
          }
          event "ThrowAway": Value Change {
            # "Change Throwaway value on EGSE"
            n75 = event-data() -> ()  [unwired: 1 in, 6 out]
            n76 = local read "Detector Resource"() -> (w124:refnum<visa-resource-name>)
            n77 = call <instrlib>:"Set ThrowAway.vi"("ThrowAway (0)"="ThrowAway", "VISA resource name"=w124) -> ()  [unwired: 8 in, 2 out]
          }
          event "DAC Value": Value Change {
            # "Change offset DAC on selected channel of detector card and store new value in detecotr data"
            n78 = event-data() -> ()  [unwired: 1 in, 6 out]
            n79 = local read "Detector Resource"() -> (w131:refnum<visa-resource-name>)
            n80 = call <instrlib>:"Set DAC.vi"("value (0)"="DAC Value", "chan (0)"="Detector", "VISA resource name"=w131) -> ()  [unwired: 7 in, 2 out]
            n81 = Index Array(array="DetectorData", index="Detector") -> (element=w130:T9)
            n82 = Bundle By Name(cluster=w130, "DAC Offset"="DAC Value") -> (w127:T9)
            n83 = Replace Array Subset(array="DetectorData", new element=w127, index="Detector") -> (w126:T3)
            n84 = local write "DetectorData"(w126) -> ()
          }
          event "Detector": Value Change {
            n85 = event-data() -> ("NewVal"=w132:u16)  [unwired: 1 in, 5 out]
            n86 = local read "DetectorData"() -> (w135:T3)
            n87 = Index Array(array=w135, index=w132) -> (element=w134:T9)
            n88 = Unbundle By Name(w134) -> ("DAC Offset"=w133:i32)
            n89 = local write "DAC Value"(w133) -> ()
          }
          event "ISweep": Value Change {
            n90 = event-data() -> ()  [unwired: 1 in, 6 out]
            n91 = case shown="True" "ISweep" {
              frame False {
              }
              frame True {
                w155 = u16 50 items=["60 Hz"=60, "50 Hz or 400 Hz"=50] ("Power Line Frequency  (60 Hz)")
                w163 = u16 1 items=["Voltage", "Current"] ("Source Mode  (0: Voltage)")
                w171 = u16 1 items=["Volts", "Current", "Resistance"] ("Function (0: Volts)")
                w174 = u16 0 items=["Volts", "Current", "Resistance"] ("Function (0: Volts)")
                w178 = u16 1 items=["Voltage", "Current"] ("Source Mode  (0: Voltage)")
                n92 = call <instrlib>:"Initialize.vi"("ID Query (True)"=FALSE, "VISA resource name"=refnum<visa-resource-name> "B2901BL") -> ("error out"=w156:errorcluster, "VISA resource name out"=w159:refnum<visa-resource-name>)  [unwired: 8 in]
                n93 = case shown="True" "SWIR/MWIR" {
                  tunnel: [1e-06 0.0001] -> w142
                  tunnel: [1e-12 1e-10] -> w138
                  tunnel: [1 ("f") 4 ("disabled index (col)")] -> w137
                  frame False {
                    # "SWIR Selected"
                  }
                  frame True {
                    # "MWIR Selected"
                  }
                }
                n94 = call <instrlib>:"Configure Power Line Frequency.vi"("error in (no error)"=w156, "Power Line Frequency  (60 Hz)"=w155, "VISA resource name"=w159) -> ("error out"=w157:errorcluster, "VISA resource name out"=w158:refnum<visa-resource-name>)  [unwired: 7 in]
                n95 = call <instrlib>:"Configure Measurement.vi"("error in (no error)"=w157, "Enable Auto Range (T:Enable)"=TRUE, "Function (0: Volts)"=w174, "VISA resource name"=w158) -> ("error out"=w169:errorcluster, "VISA resource name out"=w170:refnum<visa-resource-name>)  [unwired: 6 in]
                n96 = call <instrlib>:"Configure Measurement.vi"("error in (no error)"=w169, "Enable Auto Range (T:Enable)"=TRUE, "Function (0: Volts)"=w171, "VISA resource name"=w170) -> ("error out"=w154:errorcluster, "VISA resource name out"=w153:refnum<visa-resource-name>)  [unwired: 6 in]
                n97 = Format Into String(format string="%e", initial string=":SOUR:CURR:RANGE " ("write buffer"), w142) -> (resulting string=w139:string)  [unwired: 1 in, 1 out]
                n98 = VISA Write(VISA resource name=w153, write buffer=w139, error in (no error)=w154) -> (VISA resource name out=w152:refnum<visa-resource-name>, error out=w151:errorcluster)  [unwired: 1 out]
                n99 = local read "Detector Resource"() -> (w185:refnum<visa-resource-name>)
                n100 = call <instrlib>:"Configure Output.vi"("Source Mode  (0: Voltage)"=w178, "error in (no error)"=w151, "Output Level (0)"=0.0, "VISA resource name"=w152) -> ("error out"=w177:errorcluster, "VISA resource name out"=w176:refnum<visa-resource-name>)  [unwired: 6 in]
                n101 = case shown="True" "DecadeSweep" {
                  tunnel: [w194 w199] -> w144
                  tunnel: "NPointsPerDecade" -> [_ w198]
                  tunnel: w138 -> [_ w196]
                  frame False {
                    n102 = call-poly <vilib>:"Ramp Pattern.vi"("start"="MinCurrent", "end"="MaxCurrent", "samples"="NPoints") -> ("Ramp Pattern"=w194:dbl[])  [unwired: 7 in, 1 out]
                  }
                  frame True {
                    n103 = call "Decades125.vi"("NPointsPerDecade"=w198, "BaseUnit"=w196, "NumberDecades"=6) -> ("output array"=w199:dbl[])  [unwired: 8 in]
                  }
                }
                n104 = call <instrlib>:"Enable Output.vi"("error in (no error)"=w177, "Enable Output (T: Enable)"=TRUE ("Auto Output-Off (F: Disable)"), "VISA resource name"=w176) -> ("error out"=w167:errorcluster, "VISA resource name out"=w166:refnum<visa-resource-name>)  [unwired: 7 in]
                n105 = call <userlib>:"Wait (ms)__ogtk.vi"("error in (no error)"=w167, "milliseconds to wait"=u32 1000) -> ("error out"=w183:errorcluster)  [unwired: 8 in, 1 out]
                n106 = Initialize Array(0.0, 8 ("dimension size")) -> (w148:dbl[])
                n107 = for {
                  tunnel: w183 -> [w225]
                  tunnel: w144 -> [w217] mode=indexing
                  tunnel: [w219] -> w160
                  shift-right: [w209] -> _
                  shift-left: dbl[][] [] -> [w216]
                  tunnel: w185 -> [w218]
                  tunnel: [w224] -> w161
                  tunnel: w166 -> [w221]
                  tunnel: "SuperAverage" -> [w212]
                  tunnel: w148 -> [w211]
                  tunnel: "milliseconds stabilisation" -> [w210]
                  tunnel: w144 -> [w204]
                  tunnel: w137 -> [w200]
                  w222 = u16 1 items=["Voltage", "Current"] ("Source Mode  (0: Voltage)")
                  n108 = call <instrlib>:"Configure Output.vi"("Source Mode  (0: Voltage)"=w222, "error in (no error)"=w225, "Output Level (0)"=w217, "VISA resource name"=w221) -> ("error out"=w223:errorcluster, "VISA resource name out"=w224:refnum<visa-resource-name>)  [unwired: 6 in]
                  n109 = call <userlib>:"Wait Until Next ms Multiple__ogtk.vi"("error in (no error)"=w223, "milliseconds to wait"=w210) -> ("error out"=w220:errorcluster)  [unwired: 8 in, 1 out]
                  n110 = for {
                    N: w212 -> [_]
                    tunnel: w218 -> [w229]
                    shift-right: [w230] -> w219
                    shift-left: w220 -> [w231]
                    shift-right: [w228] -> w214
                    shift-left: w211 -> [w226]
                    n111 = call <instrlib>:"Get SCIENCE.vi"("error in (no error)"=w231, "VISA resource name"=w229) -> ("error out"=w230:errorcluster, "ScienceData"=w227:dbl[])  [unwired: 6 in, 2 out]
                    n112 = Add(x=w226, y=w227) -> (x+y=w228:dbl[])
                  }
                  n113 = Divide(x=w214, y=w212) -> (x/y=w213:dbl[])
                  n114 = Build Array (concatenate)(w217, w213) -> (w215:dbl[])
                  n115 = Build Array (concatenate)(w216, w215) -> (w209:dbl[][])
                  "Counts vs Channels" <- w209
                  n116 = Index Array(array=w209, index (col) #1=w200) -> (element #1=w203:dbl[], element #2=w202:dbl[], element #3=w201:dbl[])  [unwired: 5 in]
                  n117 = Bundle("output array"=w204, w203) -> (w208:cluster{"output array":dbl[], dbl[]})  [unwired: 1 in]
                  n118 = Bundle("output array"=w204, w202) -> (w207:cluster{"output array":dbl[], dbl[]})  [unwired: 1 in]
                  n119 = Bundle("output array"=w204, w201) -> (w206:cluster{"output array":dbl[], dbl[]})  [unwired: 1 in]
                  n120 = Build Array(w208, w207, w206) -> (→"All Channel Data":cluster{"output array":dbl[], dbl[]}[])
                }
                n121 = call <instrlib>:"Configure Output.vi"("Source Mode  (0: Voltage)"=w163, "error in (no error)"=w160, "Output Level (0)"=0.0, "VISA resource name"=w161) -> ("error out"=w164:errorcluster, "VISA resource name out"=w165:refnum<visa-resource-name>)  [unwired: 6 in]
                n122 = call <instrlib>:"Close.vi"("error in (no error)"=w164, "VISA resource name"=w165) -> ()  [unwired: 9 in, 1 out]
              }
            }
          }
          event "ISweep 2": Value Change {
            n123 = event-data() -> ()  [unwired: 1 in, 6 out]
            n124 = case shown="True" "ISweep 2" {
              frame False {
              }
              frame True {
                w261 = u16 3 items=["1", "3", "9", "20"] ("NPointsPerDecade")
                n125 = case shown="False" "SWIR/MWIR 2" {
                  tunnel: [1 ("f") 4 ("f")] -> w259
                  tunnel: [w284 w289] -> w249
                  tunnel: [w285 w290] -> w252
                  tunnel: [1e-11 1e-09 ("x")] -> w257
                  tunnel: 98902.0 ("x") -> [_ w290]
                  tunnel: 9991340.0 -> [w285 _]
                  tunnel: refnum<k21> "Dev0/Ao5" ("physical channels") -> [w283 w289]
                  tunnel: refnum<k21> "Dev0/Ao3" ("physical channels") -> [w284 w288]
                  tunnel: [w283 w288] -> w242
                  frame False {
                    # "SWIR"
                  }
                  frame True {
                    # "MWIR"
                  }
                }
                n126 = call-poly <instrlib>:"ULx Create Virtual Channel.vi"("maximum value"=10.0, "minimum value"=-10.0, "physical channels"=w242) -> ("task out"=w245:refnum<k24>, "error out"=w248:errorcluster)  [unwired: 11 in]
                n127 = call-poly <instrlib>:"ULx Write.vi"("task in"=w245, "data"="Other Channel Forcing", "timeout"=100.0, "error in"=w248) -> ("task out"=w239:refnum<k24>, "error out"=w241:errorcluster)  [unwired: 9 in, 1 out]
                n128 = call-poly <instrlib>:"ULx Create Virtual Channel.vi"("maximum value"=10.0, "minimum value"=-10.0, "physical channels"=w249, "error in"=w241) -> ("task out"=w272:refnum<k24>, "error out"=w269:errorcluster)  [unwired: 10 in]
                n129 = call "Decades125.vi"("NPointsPerDecade"=w261, "BaseUnit"=1.0, "NumberDecades"=5) -> ("output array"=w258:dbl[])  [unwired: 8 in]
                n130 = Multiply(x=w257, y=w258) -> (x*y=w256:dbl[])
                n131 = call-poly <instrlib>:"ULx Write.vi"("task in"=w272, "data"=0.0, "timeout"=100.0, "error in"=w269) -> ("task out"=w268:refnum<k24>, "error out"=w267:errorcluster)  [unwired: 9 in, 1 out]
                n132 = local read "Detector Resource"() -> (w282:refnum<visa-resource-name>)
                n133 = Multiply(x=w252, y=w256) -> (x*y=w255:dbl[])
                n134 = call <userlib>:"Wait (ms)__ogtk.vi"("error in (no error)"=w267, "milliseconds to wait"=u32 1000) -> ("error out"=w281:errorcluster)  [unwired: 8 in, 1 out]
                n135 = Initialize Array(0.0, 8 ("dimension size")) -> (w277:dbl[])
                n136 = for {
                  tunnel: w281 -> [w300]
                  tunnel: [w317] -> w234
                  shift-right: [w309] -> _
                  shift-left: dbl[][] [] -> [w315]
                  tunnel: w282 -> [w316]
                  tunnel: [w298] -> w264
                  tunnel: w277 -> [w311]
                  tunnel: "milliseconds stabilisation 2" -> [w310]
                  tunnel: w259 -> [w301]
                  tunnel: w268 -> [w299]
                  tunnel: w256 -> [w295]
                  tunnel: w256 -> [w294] mode=indexing
                  tunnel: w255 -> [w293] mode=indexing
                  n137 = call-poly <instrlib>:"ULx Write.vi"("task in"=w299, "data"=w293, "error in"=w300) -> ("task out"=w298:refnum<k24>, "error out"=w297:errorcluster)  [unwired: 10 in, 1 out]
                  n138 = call <userlib>:"Wait Until Next ms Multiple__ogtk.vi"("error in (no error)"=w297, "milliseconds to wait"=w310) -> ("error out"=w318:errorcluster)  [unwired: 8 in, 1 out]
                  n139 = for {
                    N: "SuperAvg" -> [_]
                    tunnel: w316 -> [w322]
                    shift-right: [w323] -> w317
                    shift-left: w318 -> [w324]
                    shift-right: [w321] -> w313
                    shift-left: w311 -> [w319]
                    n140 = call <instrlib>:"Get SCIENCE.vi"("error in (no error)"=w324, "VISA resource name"=w322) -> ("error out"=w323:errorcluster, "ScienceData"=w320:dbl[])  [unwired: 6 in, 2 out]
                    n141 = Add(x=w319, y=w320) -> (x+y=w321:dbl[])
                  }
                  n142 = Divide(x=w313, y="SuperAvg") -> (x/y=w312:dbl[])
                  n143 = Build Array (concatenate)(w294, w312) -> (w314:dbl[])
                  n144 = Build Array (concatenate)(w315, w314) -> (w309:dbl[][])
                  "Counts vs Channels 2" <- w309
                  n145 = Index Array(array=w309, index (col) #1=w301) -> (element #1=w304:dbl[], element #2=w303:dbl[], element #3=w302:dbl[])  [unwired: 5 in]
                  n146 = Bundle(w295, w304) -> (w308:cluster{dbl[], dbl[]})  [unwired: 1 in]
                  n147 = Bundle(w295, w303) -> (w307:cluster{dbl[], dbl[]})  [unwired: 1 in]
                  n148 = Bundle(w295, w302) -> (w306:cluster{dbl[], dbl[]})  [unwired: 1 in]
                  n149 = Build Array(w308, w307, w306) -> (→"All Channel Data 2":cluster{dbl[], dbl[]}[])
                }
                n150 = call-poly <instrlib>:"ULx Write.vi"("task in"=w239, "data"=0.0, "error in"=w234) -> ("task out"=w236:refnum<k24>, "error out"=w235:errorcluster)  [unwired: 10 in, 1 out]
                n151 = call <instrlib>:"ULx Clear Task.vi"("task in"=w236, "error in"=w235) -> ("error out"=w233:errorcluster)  [unwired: 13 in]
                n152 = call-poly <instrlib>:"ULx Write.vi"("task in"=w264, "data"=0.0, "timeout"=100.0, "error in"=w233) -> ("task out"=w238:refnum<k24>, "error out"=w237:errorcluster)  [unwired: 9 in, 1 out]
                n153 = call <instrlib>:"ULx Clear Task.vi"("task in"=w238, "error in"=w237) -> ()  [unwired: 13 in, 1 out]
              }
            }
          }
          event "Heater": Value Change {
            n154 = event-data() -> ()  [unwired: 1 in, 6 out]
            n155 = local read "Detector Resource"() -> (w325:refnum<visa-resource-name>)
            n156 = call "Set Heater.vi"("Power (0)"="Heater", "VISA resource name"=w325) -> ()  [unwired: 8 in, 2 out]
          }
          event "ExportData": Value Change {
            n157 = event-data() -> ()  [unwired: 1 in, 6 out]
            n158 = call "File Dialog2"("prompt"="Give name for save file", "pattern (all files)"="*.txt", "pattern label"="CSV text Files") -> ("selected path"=w327:path, "cancelled"=w328:bool)  [unwired: 9 in, 2 out]
            n159 = case shown="False" w328 {
              tunnel: w327 -> [w332 _]
              frame False {
                n160 = local read "Counts vs Channels 2"() -> (w333:dbl[][])
                n161 = call-poly <vilib>:"Write Delimited Spreadsheet.vi"("file path (dialog if empty)"=w332, "format (%.3f)"="%.4g", "2D data"=w333) -> ()  [unwired: 11 in, 2 out]
              }
              frame True {
              }
            }
          }
          event "SweepLight": Value Change {
            n162 = event-data() -> ()  [unwired: 1 in, 6 out]
            n163 = case shown="True" "SweepLight" {
              frame False {
              }
              frame True {
                w352 = dbl[] []
                n164 = disable-structure shown="Disabled" {
                  disable-tunnel: [w362 _] -> w353
                  frame Disabled {
                    n165 = call "Keithley 648X Series SetupAcquisition.vi"("VISA resource name"=refnum<visa-resource-name> "Picoammeter") -> ("VISA resource name out"=w362:refnum<visa-resource-name>)  [unwired: 8 in, 1 out]
                  }
                  frame Enabled {
                  }
                }
                n166 = local read "Detector Resource"() -> (w360:refnum<visa-resource-name>)
                n167 = local read "Oversample"() -> (w361:i32)
                n168 = call-poly <vilib>:"Ramp Pattern.vi"("start"="Modulation Min", "end"="Modulation Max", "samples"="Modulation Steps") -> ("Ramp Pattern"=w356:dbl[])  [unwired: 7 in, 1 out]
                n169 = call <instrlib>:"Set DAC.vi"("value (0)"="DAC", "chan (0)"="Detector 7", "VISA resource name"=w360) -> ("error out"=w351:errorcluster, "VISA resource name out"=w359:refnum<visa-resource-name>)  [unwired: 7 in]
                n170 = call <instrlib>:"ULx Create Channel (AO-Voltage-Basic).vi"("maximum value"=5.0, "minimum value"=0.0, "physical channels"=refnum<k21> "Dev0/Ao0", "error in"=w351) -> ("task out"=w346:refnum<k24>, "error out"=w345:errorcluster)  [unwired: 10 in]
                n171 = call <instrlib>:"ULx Write (Analog 1D DBL 1Chan 1Samp).vi"("task in"=w346, "data"="Modulation Min", "error in"=w345) -> ("task out"=w347:refnum<k24>, "error out"=w342:errorcluster)  [unwired: 10 in, 1 out]
                n172 = call <userlib>:"Wait (ms)__ogtk.vi"("error in (no error)"=w342, "milliseconds to wait"=u32 1000) -> ("error out"=w343:errorcluster)  [unwired: 8 in, 1 out]
                n173 = for {
                  tunnel: w343 -> [w392]
                  tunnel: [w391] -> w337
                  tunnel: [w373] -> w339
                  shift-right: [w386] -> _
                  shift-left: w352 -> [w388]
                  tunnel: w359 -> [w385]
                  shift-right: [w381] -> _
                  shift-left: w352 -> [w383]
                  shift-right: [w380] -> _
                  shift-left: w352 -> [w382]
                  tunnel: w361 -> [w375]
                  tunnel: "Detector 7" -> [w374]
                  tunnel: w356 -> [w366] mode=indexing
                  tunnel: w353 -> [w372]
                  shift-right: [w368] -> _
                  shift-left: w352 -> [w369]
                  tunnel: w347 -> [w367]
                  stop <- "Abort 2" stop-if-true
                  n174 = call <instrlib>:"ULx Write (Analog 1D DBL 1Chan 1Samp).vi"("task in"=w367, "data"=w366, "error in"=w392) -> ("task out"=w391:refnum<k24>, "error out"=w390:errorcluster)  [unwired: 10 in, 1 out]
                  n175 = call <instrlib>:"Get ADC.vi"("Gain"="Gain 2", "Detector"=w374, "error in (no error)"=w390, "VISA resource name"=w385) -> ("error out"=w384:errorcluster, "output"=w387:i32)  [unwired: 5 in, 1 out]
                  n176 = Divide(x=w387, y=w375) -> (x/y=w364:dbl)
                  n177 = Build Array (concatenate)(w383, w364) -> (w381:dbl[])
                  n178 = Build Array (concatenate)(w388, w364) -> (w386:dbl[])
                  n179 = Build Array (concatenate)(w382, w364) -> (w380:dbl[])
                  n180 = call <instrlib>:"Measure Current.vi"("VISA resource name"=w372, "error in (no error)"=w384) -> ("Measurement"=w370:dbl, "error out"=w373:errorcluster)  [unwired: 11 in, 1 out]
                  n181 = Negate(x=w370) -> (-x=w365:dbl)
                  n182 = Build Array (concatenate)(w369, w365) -> (w368:dbl[])
                  n183 = Bundle(w368, w386) -> (w379:cluster{dbl[], dbl[]})  [unwired: 1 in]
                  n184 = Bundle(w368, w381) -> (w378:cluster{dbl[], dbl[]})  [unwired: 1 in]
                  n185 = Bundle(w368, w380) -> (w377:cluster{dbl[], dbl[]})  [unwired: 1 in]
                  n186 = Build Array(w379, w378, w377) -> (→"Output vs Light":cluster{dbl[], dbl[]}[])
                }
                n187 = call <instrlib>:"ULx Write (Analog 1D DBL 1Chan 1Samp).vi"("task in"=w337, "data"=0.0, "error in"=w339) -> ("task out"=w338:refnum<k24>, "error out"=w340:errorcluster)  [unwired: 10 in, 1 out]
                n188 = call <instrlib>:"ULx Clear Task.vi"("task in"=w338, "error in"=w340) -> ()  [unwired: 13 in, 1 out]
              }
            }
          }
          event "SweepVDAC": Value Change {
            n189 = event-data() -> ()  [unwired: 1 in, 6 out]
            n190 = case shown="True" "SweepVDAC" {
              frame False {
              }
              frame True {
                w406 = u16 1 items=["Voltage", "Current"] ("Source Mode  (0: Voltage)")
                w408 = dbl[] []
                w421 = u16 1 items=["Voltage", "Current"] ("Source Mode  (0: Voltage)")
                w425 = u16 1 items=["Volts", "Current", "Resistance"] ("Function (0: Volts)")
                w427 = u16 0 items=["Volts", "Current", "Resistance"] ("Function (0: Volts)")
                n191 = call <instrlib>:"Initialize.vi"("ID Query (True)"=FALSE, "VISA resource name"="Current source") -> ("error out"=w413:errorcluster, "VISA resource name out"=w414:refnum<visa-resource-name>)  [unwired: 8 in]
                n192 = call <instrlib>:"Configure Measurement.vi"("error in (no error)"=w413, "Enable Auto Range (T:Enable)"=TRUE, "Function (0: Volts)"=w427, "VISA resource name"=w414) -> ("error out"=w428:errorcluster, "VISA resource name out"=w429:refnum<visa-resource-name>)  [unwired: 6 in]
                n193 = call <instrlib>:"Configure Measurement.vi"("Manual Range (1.0)"=1e-07, "error in (no error)"=w428, "Enable Auto Range (T:Enable)"=FALSE, "Function (0: Volts)"=w425, "VISA resource name"=w429) -> ("error out"=w423:errorcluster, "VISA resource name out"=w422:refnum<visa-resource-name>)  [unwired: 5 in]
                n194 = call-poly <vilib>:"Ramp Pattern.vi"("start"="VDAC Min", "end"="VDAC Max", "delta"="VDAC Step") -> ("Ramp Pattern"=w410:dbl[])  [unwired: 6 in, 2 out]
                n195 = local read "Oversample"() -> (w407:i32)
                n196 = local read "Detector Resource"() -> (w409:refnum<visa-resource-name>)
                n197 = call <instrlib>:"Configure Output.vi"("Source Mode  (0: Voltage)"=w421, "error in (no error)"=w423, "Output Level (0)"="ISource", "VISA resource name"=w422) -> ("error out"=w420:errorcluster, "VISA resource name out"=w419:refnum<visa-resource-name>)  [unwired: 6 in]
                n198 = call <instrlib>:"Enable Output.vi"("error in (no error)"=w420, "Enable Output (T: Enable)"=TRUE, "VISA resource name"=w419) -> ("error out"=w416:errorcluster, "VISA resource name out"=w417:refnum<visa-resource-name>)  [unwired: 7 in]
                n199 = for {
                  tunnel: w417 -> [w433]
                  tunnel: w416 -> [w464]
                  tunnel: w410 -> [w463] mode=indexing
                  tunnel: [w433] -> w405
                  tunnel: [w455] -> w403
                  shift-right: [w458] -> _
                  shift-left: w408 -> [w460]
                  tunnel: w410 -> [w446]
                  tunnel: w409 -> [w432]
                  shift-right: [w448] -> _
                  shift-left: w408 -> [w450]
                  shift-right: [w447] -> _
                  shift-left: w408 -> [w449]
                  tunnel: w407 -> [w436]
                  tunnel: "Detector 5" -> [w434]
                  stop <- "Abort SweepVDAC" stop-if-true
                  w451 = u16 2 items=["High", "Med", "Low"] ("Gain")
                  w452 = u16 1 items=["High", "Med", "Low"] ("Gain")
                  w461 = u16 0 items=["High", "Med", "Low"] ("Gain")
                  n200 = call <instrlib>:"Set DAC.vi"("error in (no error)"=w464, "value (0)"=w463, "chan (0)"=w434, "VISA resource name"=w432) -> ("error out"=w462:errorcluster, "VISA resource name out"=w431:refnum<visa-resource-name>)  [unwired: 6 in]
                  n201 = call <instrlib>:"Get ADC.vi"("Gain"=w461, "Detector"=w434, "error in (no error)"=w462, "VISA resource name"=w431) -> ("error out"=w457:errorcluster, "output"=w459:i32, "VISA resource name out"=w454:refnum<visa-resource-name>)  [unwired: 5 in]
                  n202 = Divide(x=w459, y=w436) -> (x/y=w440:dbl)
                  n203 = call <instrlib>:"Get ADC.vi"("Gain"=w452, "Detector"=w434, "error in (no error)"=w457, "VISA resource name"=w454) -> ("error out"=w456:errorcluster, "output"=w439:i32, "VISA resource name out"=w453:refnum<visa-resource-name>)  [unwired: 5 in]
                  n204 = Divide(x=w439, y=w436) -> (x/y=w438:dbl)
                  n205 = call <instrlib>:"Get ADC.vi"("Gain"=w451, "Detector"=w434, "error in (no error)"=w456, "VISA resource name"=w453) -> ("error out"=w455:errorcluster, "output"=w435:i32)  [unwired: 5 in, 1 out]
                  n206 = Divide(x=w435, y=w436) -> (x/y=w437:dbl)
                  n207 = Build Array (concatenate)(w450, w438) -> (w448:dbl[])
                  n208 = Build Array (concatenate)(w460, w440) -> (w458:dbl[])
                  n209 = Build Array (concatenate)(w449, w437) -> (w447:dbl[])
                  n210 = Bundle("Ramp Pattern"=w446, w458) -> (w445:cluster{"Ramp Pattern":dbl[], dbl[]})  [unwired: 1 in]
                  n211 = Bundle("Ramp Pattern"=w446, w448) -> (w444:cluster{"Ramp Pattern":dbl[], dbl[]})  [unwired: 1 in]
                  n212 = Bundle("Ramp Pattern"=w446, w447) -> (w443:cluster{"Ramp Pattern":dbl[], dbl[]})  [unwired: 1 in]
                  n213 = Build Array(w445, w444, w443) -> (→"VDAC Sweep":cluster{"Ramp Pattern":dbl[], dbl[]}[])
                }
                n214 = call <instrlib>:"Configure Output.vi"("Source Mode  (0: Voltage)"=w406, "error in (no error)"=w403, "Output Level (0)"=0.0, "VISA resource name"=w405) -> ("error out"=w402:errorcluster, "VISA resource name out"=w404:refnum<visa-resource-name>)  [unwired: 6 in]
                n215 = call <instrlib>:"Enable Output.vi"("error in (no error)"=w402, "Enable Output (T: Enable)"=FALSE, "VISA resource name"=w404) -> ("error out"=w412:errorcluster, "VISA resource name out"=w411:refnum<visa-resource-name>)  [unwired: 7 in]
                n216 = call <instrlib>:"Close.vi"("error in (no error)"=w412, "VISA resource name"=w411) -> ()  [unwired: 9 in, 1 out]
              }
            }
          }
          event "Find Offset": Value Change {
            n217 = event-data() -> ()  [unwired: 1 in, 6 out]
            n218 = local read "Detector Resource"() -> (w471:refnum<visa-resource-name>)
            n219 = property on="Searching..." class="Bool (strict)"("Value"=TRUE ("Searching...")) -> (error out=w477:errorcluster)  [unwired: 2 in, 1 out]
            n220 = local read "Detector"() -> (w472:u16)
            n221 = while {
              shift-right: [w489] -> _
              shift-left: 4095 -> [w484]
              shift-right: [w488] -> _
              shift-left: 1 -> [w485]
              tunnel: w477 -> [w494]
              tunnel: [w480] -> w474
              tunnel: w472 -> [w491]
              tunnel: w471 -> [w490]
              tunnel: [w487] -> w469 mode=indexing
              tunnel: [w486] -> w470 mode=indexing
              tunnel: [w479] -> w468 mode=indexing
              tunnel: [w482] -> w465 mode=indexing
              stop <- w495 stop-if-true
              n222 = Subtract(x=w484, y=w485) -> (x-y=w497:i32)
              n223 = Absolute Value(x=w497) -> (abs(x)=w493:i32)
              n224 = Less Or Equal?(x=w493, y=1) -> (x <= y?=w496:bool)
              n225 = case shown="False" w496 {
                tunnel: w484 -> [w510 w546]
                tunnel: w485 -> [w509 w548]
                tunnel: [w508 w548] -> w488
                tunnel: [w511 TRUE] -> w495
                tunnel: w494 -> [w522 _]
                tunnel: [w506 w546] -> w489
                tunnel: [w505 _] -> w481
                tunnel: w491 -> [w503 _]
                tunnel: w490 -> [w502 _]
                tunnel: [w498 w546] -> w483
                frame False {
                  # "Not there yet."
                  n226 = Add(x=w510, y=w509) -> (x+y=w524:i32)
                  n227 = Quotient & Remainder(x=w524, y=2) -> (floor(x/y)=w498:i32)  [unwired: 1 out]
                  n228 = local write "DAC Value"(w498) -> ()
                  n229 = call <instrlib>:"Set DAC.vi"("error in (no error)"=w522, "value (0)"=w498, "chan (0)"=w503, "VISA resource name"=w502) -> ("error out"=w521:errorcluster, "VISA resource name out"=w518:refnum<visa-resource-name>)  [unwired: 6 in]
                  n230 = call <userlib>:"Wait (ms)__ogtk.vi"("error in (no error)"=w521, "milliseconds to wait"=u32 5) -> ("error out"=w519:errorcluster)  [unwired: 8 in, 1 out]
                  n231 = local read "Oversample"() -> (w517:i32)
                  n232 = for {
                    N: "Avg" -> [_]
                    tunnel: w518 -> [w529]
                    tunnel: [w527] -> w516 mode=indexing
                    tunnel: w503 -> [w525]
                    shift-right: [w526] -> w505
                    shift-left: w519 -> [w530]
                    w528 = u16 0 items=["High", "Med", "Low"] ("Gain")
                    n233 = call <instrlib>:"Get ADC.vi"("Gain"=w528, "Detector"=w525, "error in (no error)"=w530, "VISA resource name"=w529) -> ("error out"=w526:errorcluster, "output"=w527:i32)  [unwired: 5 in, 1 out]
                  }
                  n234 = Add Array Elements(numeric array=w516) -> (sum=w501:i32)
                  n235 = Divide(x=w501, y="Avg") -> (x/y=w500:dbl)
                  n236 = Divide(x=w500, y=w517) -> (x/y=w504:dbl)
                  n237 = Subtract(x=w504, y="Target Counts") -> (x-y=w507:dbl)
                  n238 = local write "Counts"(w504) -> ()
                  n239 = Absolute Value(x=w507) -> (abs(x)=w514:dbl)
                  n240 = Less?(x=w514, y="Tolerance") -> (x < y?=w512:bool)
                  n241 = case shown="True" w512 {
                    tunnel: [FALSE TRUE] -> w511
                    tunnel: w498 -> [w534 w544]
                    tunnel: w510 -> [w535 w543]
                    tunnel: w509 -> [w533 _]
                    tunnel: [w531 w544] -> w508
                    tunnel: w507 -> [w537 _]
                    tunnel: [w532 w543] -> w506
                    frame False {
                      # "Not there, so examine difference\nbetween target and reading"
                      n242 = Greater Than 0?(x=w537) -> (x > 0?=w536:bool)
                      n243 = case shown="False" w536 {
                        tunnel: w535 -> [_ w542]
                        tunnel: w534 -> [w540 w541]
                        tunnel: w533 -> [w539 _]
                        tunnel: [w540 w542] -> w532
                        tunnel: [w539 w541] -> w531
                        frame False {
                          # "Reading is below target, so next DAC vaue will be below midpoint"
                        }
                        frame True {
                          # "If reading is above target, then next DAC value will be above mid"
                        }
                      }
                    }
                    frame True {
                      # "Within tolerance, so finish"
                    }
                  }
                }
                frame True {
                  # "DAC Values identical so finish"
                }
              }
              n244 = property on="Counts" class="WFChart (strict)"(error in=w481) -> (error out=w480:errorcluster, "Value"=w479:dbl)  [unwired: 1 in, 1 out]
              n245 = To Double Precision Float(number=w484) -> (double precision float=w487:dbl)
              n246 = To Double Precision Float(number=w483) -> (double precision float=w482:dbl)
              n247 = To Double Precision Float(number=w485) -> (double precision float=w486:dbl)
            }
            n248 = Build Array(w470, w469, w465, w468) -> (w467:dbl[][])
            n249 = property on="Searching..." class="Bool (strict)"(error in=w474, "Value"=FALSE ("Searching...")) -> ()  [unwired: 1 in, 2 out]
            n250 = Transpose 2D Array(2D array=w467) -> (transposed array=→"Searching":dbl[][])
          }
          event "Export Button": Value Change {
            n251 = event-data() -> ()  [unwired: 1 in, 6 out]
            n252 = call "File Dialog"("prompt"="Give name for save file", "pattern (all files)"="*.txt", "pattern label"="CSV Text files") -> ("selected path"=w549:path, "cancelled"=w550:bool)  [unwired: 9 in, 2 out]
            n253 = case shown="False" w550 {
              tunnel: w549 -> [w556 _]
              frame False {
                n254 = local read "Counts vs Channels"() -> (w555:dbl[][])
                n255 = call-poly <vilib>:"Write Delimited Spreadsheet.vi"("file path (dialog if empty)"=w556, "format (%.3f)"="%.4g", "2D data"=w555) -> ()  [unwired: 11 in, 2 out]
              }
              frame True {
              }
            }
          }
          event "NoiseSweep": Value Change {
            w570 = u16 3 items=["1", "3", "9", "20"] ("NPointsPerDecade")
            w578 = u16 0 items=["Sine", "Square", "Ramp", "Trangle", "Pulse", "Noise"] ("Waveform Function (0: Sine)")
            n256 = event-data() -> ()  [unwired: 1 in, 6 out]
            n257 = call <instrlib>:"Initialize.vi"("VISA resource name"=refnum<visa-resource-name> "TG5011A") -> ("error out"=w579:errorcluster, "VISA resource name out"=w580:refnum<visa-resource-name>)  [unwired: 9 in]
            n258 = local read "Detector VISA"() -> (w563:refnum<visa-resource-name>)
            n259 = call <instrlib>:"Configure Standard Waveform.vi"("Frequency (1000 Hz)"=1000.0, "error in (no error)"=w579, "Amplitude (1.0 Vpp)"=10.0, "Waveform Function (0: Sine)"=w578, "VISA resource name"=w580) -> ("error out"=w574:errorcluster, "VISA resource name out"=w575:refnum<visa-resource-name>)  [unwired: 5 in]
            n260 = call "Decades125.vi"("NPointsPerDecade"=w570, "BaseUnit"=1.0, "NumberDecades"=4) -> ("output array"=w562:dbl[])  [unwired: 8 in]
            n261 = call <instrlib>:"Enable Output.vi"("Enable Output (T: Enable)"=TRUE, "error in (no error)"=w574, "VISA resource name"=w575) -> ("error out"=w560:errorcluster, "VISA resource name out"=w569:refnum<visa-resource-name>)  [unwired: 7 in]
            n262 = call <userlib>:"Wait (ms)__ogtk.vi"("error in (no error)"=w560, "milliseconds to wait"=u32 1000) -> ("error out"=w559:errorcluster)  [unwired: 8 in, 1 out]
            n263 = for {
              tunnel: w562 -> [w598] mode=indexing
              tunnel: w569 -> [w600]
              tunnel: w559 -> [w599]
              tunnel: [w583] -> w566
              tunnel: [w597] -> w567
              tunnel: w563 -> [w595]
              tunnel: w562 -> [w585]
              shift-right: [w584] -> _
              shift-left: dbl[] [] -> [w588]
              tunnel: "Channel" -> [w582]
              w602 = u16 0 items=["Sine", "Square", "Ramp", "Trangle", "Pulse", "Noise"] ("Waveform Function (0: Sine)")
              n264 = call <instrlib>:"Configure Standard Waveform.vi"("Frequency (1000 Hz)"=w598, "error in (no error)"=w599, "Amplitude (1.0 Vpp)"=10.0, "Waveform Function (0: Sine)"=w602, "VISA resource name"=w600) -> ("error out"=w594:errorcluster, "VISA resource name out"=w597:refnum<visa-resource-name>)  [unwired: 5 in]
              n265 = for {
                N: "SamplesToAverage" -> [_]
                tunnel: w595 -> [w608]
                tunnel: w594 -> [w607]
                tunnel: [w605] -> w593 mode=indexing
                tunnel: [w604] -> w591
                tunnel: w582 -> [w603]
                n266 = call <instrlib>:"Get SCIENCE.vi"("error in (no error)"=w607, "VISA resource name"=w608) -> ("error out"=w604:errorcluster, "ScienceData"=w606:dbl[])  [unwired: 6 in, 2 out]
                n267 = Index Array(array=w606, index=w603) -> (element=w605:dbl)
              }
              n268 = Bundle By Name("Y"=w593) -> (w592:waveform(dbl))  [unwired: 1 in]
              n269 = call-poly <vilib>:"Amplitude and Levels.vi"("error in (no error)"=w591, "signal in"=w592) -> ("error out"=w583:errorcluster, "low state level"=w590:dbl, "high state level"=w589:dbl)  [unwired: 6 in, 1 out]
              n270 = Subtract(x=w589, y=w590) -> (x-y=w587:dbl)
              n271 = Build Array (concatenate)(w588, w587) -> (w584:dbl[])
              n272 = Bundle("output array"=w585, w584) -> (→"XY Graph":cluster{"output array":dbl[], dbl[]})  [unwired: 1 in]
            }
            n273 = call <instrlib>:"Enable Output.vi"("Enable Output (T: Enable)"=FALSE, "error in (no error)"=w566, "VISA resource name"=w567) -> ("error out"=w565:errorcluster, "VISA resource name out"=w564:refnum<visa-resource-name>)  [unwired: 7 in]
            n274 = call <instrlib>:"Close.vi"("error in (no error)"=w565, "VISA resource name"=w564) -> ()  [unwired: 9 in, 1 out]
          }
          event "Exit": Value Change {
            # "If stage is connected, go to reference position and then exit"
            n275 = event-data() -> ()  [unwired: 1 in, 6 out]
          }
          event Panel Close? {
            # "Discard \"Panel Close?\" event\n\nto leave program through\n graceful route"
            # "NOTE:\nMake sure not to use the red \"Abort Execution\" button in the\nLabVIEW menu to abort the application execution.\nDoing so will not close the device connection with the consequence that\na re-open after the next application start will fail."
            # "\"Panel Close\" (\"X\") was clicked by the user:\nWe discard the close command and set an \"exit\" flag. This gives us the change to proper disconnect the device and clean up the application before closing the window."
            # "Trap \"Panel Close\" instruction and exit program gracefully"
            n276 = event-data() -> ()  [unwired: 1 in, 4 out]
            n277 = local write "exit"(TRUE ("exit")) -> ()
            n278 = event-data("Discard?"=TRUE) -> ()  [unwired: 1 in, 1 out]
          }
        }
      }
    }
    frame #2 {
      # "Also power off and close detector SCPI EGSE"
      # "Cleanup and Shutdown"
      n279 = local read "Detector Resource"() -> (w616:refnum<visa-resource-name>)
      n280 = call <instrlib>:"Set Power.vi"("Power (0)"=FALSE, "VISA resource name"=w616) -> ("error out"=w613:errorcluster, "VISA resource name out"=w617:refnum<visa-resource-name>)  [unwired: 8 in]
      n281 = property on="Power" class="Bool (strict)"(error in=w613, "Value"=FALSE ("Power")) -> (error out=w614:errorcluster)  [unwired: 1 in, 1 out]
      n282 = call <instrlib>:"Close.vi"("error in (no error)"=w614, "VISA resource name"=w617) -> ()  [unwired: 9 in, 1 out]
    }
  }
  "error out" <- w1
